vi "虛擬儀控期末專題R09543010張哲睿主程式.vi"() -> ()   [LabVIEW 2014]
uses:
  <vilib>/Math Plots/3D Math Plots/3D Pie/3D Pie XCtrl/3D Pie.xctl
  <vilib>/Math Plots/3D Math Plots/3D Pie/3D Pie Datatype/Public/Plot Helper (Vector).vi
  <vilib>/Math Plots/3D Math Plots/3D Pie/3D Pie Datatype/3D Pie Datatype.lvclass
panel:
  in  "再感染機率":dbl=20.0 format="%#_13g%%"
  out "3D Pie":refnum<class "3D Plot Datatype.lvclass">[](xcontrol)
  out "P10 Infeted":enum16{"Infected", "Uninfected"}(ring)
  out "P9 Infeted?":enum16{"Infected", "Uninfected"}(ring)
  out "P8 Infeted?":enum16{"Infected", "Uninfected"}(ring)
  out "P7 Infeted?":enum16{"Infected", "Uninfected"}(ring)
  out "P6 Infeted?":enum16{"Infected", "Uninfected"}(ring)
  out "P5 Infeted?":enum16{"Infected", "Uninfected"}(ring)
  out "P4 Infeted?":enum16{"Infected", "Uninfected"}(ring)
  out "P3 Infeted?":enum16{"Infected", "Uninfected"}(ring)
  out "P2 Infeted?":enum16{"Infected", "Uninfected"}(ring)
  out "P1 Infeted?":enum16{"Infected", "Uninfected"}(ring)
  in  "死亡率":dbl=50.0 format="%#_g%%"
  in  "陰轉陽率":dbl=50.0 format="%#_g%%"
  out "Alive? P10":enum16{"Alive", "Dead"}(ring)
  out "Alive? P9":enum16{"Alive", "Dead"}(ring)
  out "Alive? P8":enum16{"Alive", "Dead"}(ring)
  out "Alive? P7":enum16{"Alive", "Dead"}(ring)
  out "Alive? P6":enum16{"Alive", "Dead"}(ring)
  out "Alive? P5":enum16{"Alive", "Dead"}(ring)
  out "Alive? P4":enum16{"Alive", "Dead"}(ring)
  out "Alive? P3":enum16{"Alive", "Dead"}(ring)
  out "Alive? P2":enum16{"Alive", "Dead"}(ring)
  out "Alive? P1":enum16{"Alive", "Dead"}(ring)
  in  "stop":bool
  out "Y":i32[](array[numeric])
  out "X":i32[](array[numeric])
  out "Numeric":i32
  out "P1":bool
  in  "Bound right":dbl=300.0
  in  "Bound bottom":dbl=300.0
  out "State":T1(ring)
  out "P2":bool
  out "State 2":T1(ring)
  out "State 3":T1(ring)
  out "P3":bool
  out "P4":bool
  out "State 4":T1(ring)
  out "State 5":T1(ring)
  out "P5":bool
  out "State 6":T1(ring)
  out "P6":bool
  out "State 7":T1(ring)
  out "P7":bool
  out "State 8":T1(ring)
  out "State 9":T1(ring)
  out "State 10":T1(ring)
  out "P8":bool
  out "P9":bool
  out "P10":bool
  # "註:因內建3D Pie Chart的問題，偶爾打開VI時Pie Chart鐘百分比符號\n無法正常顯示，檔案重開一次即可解決問題"
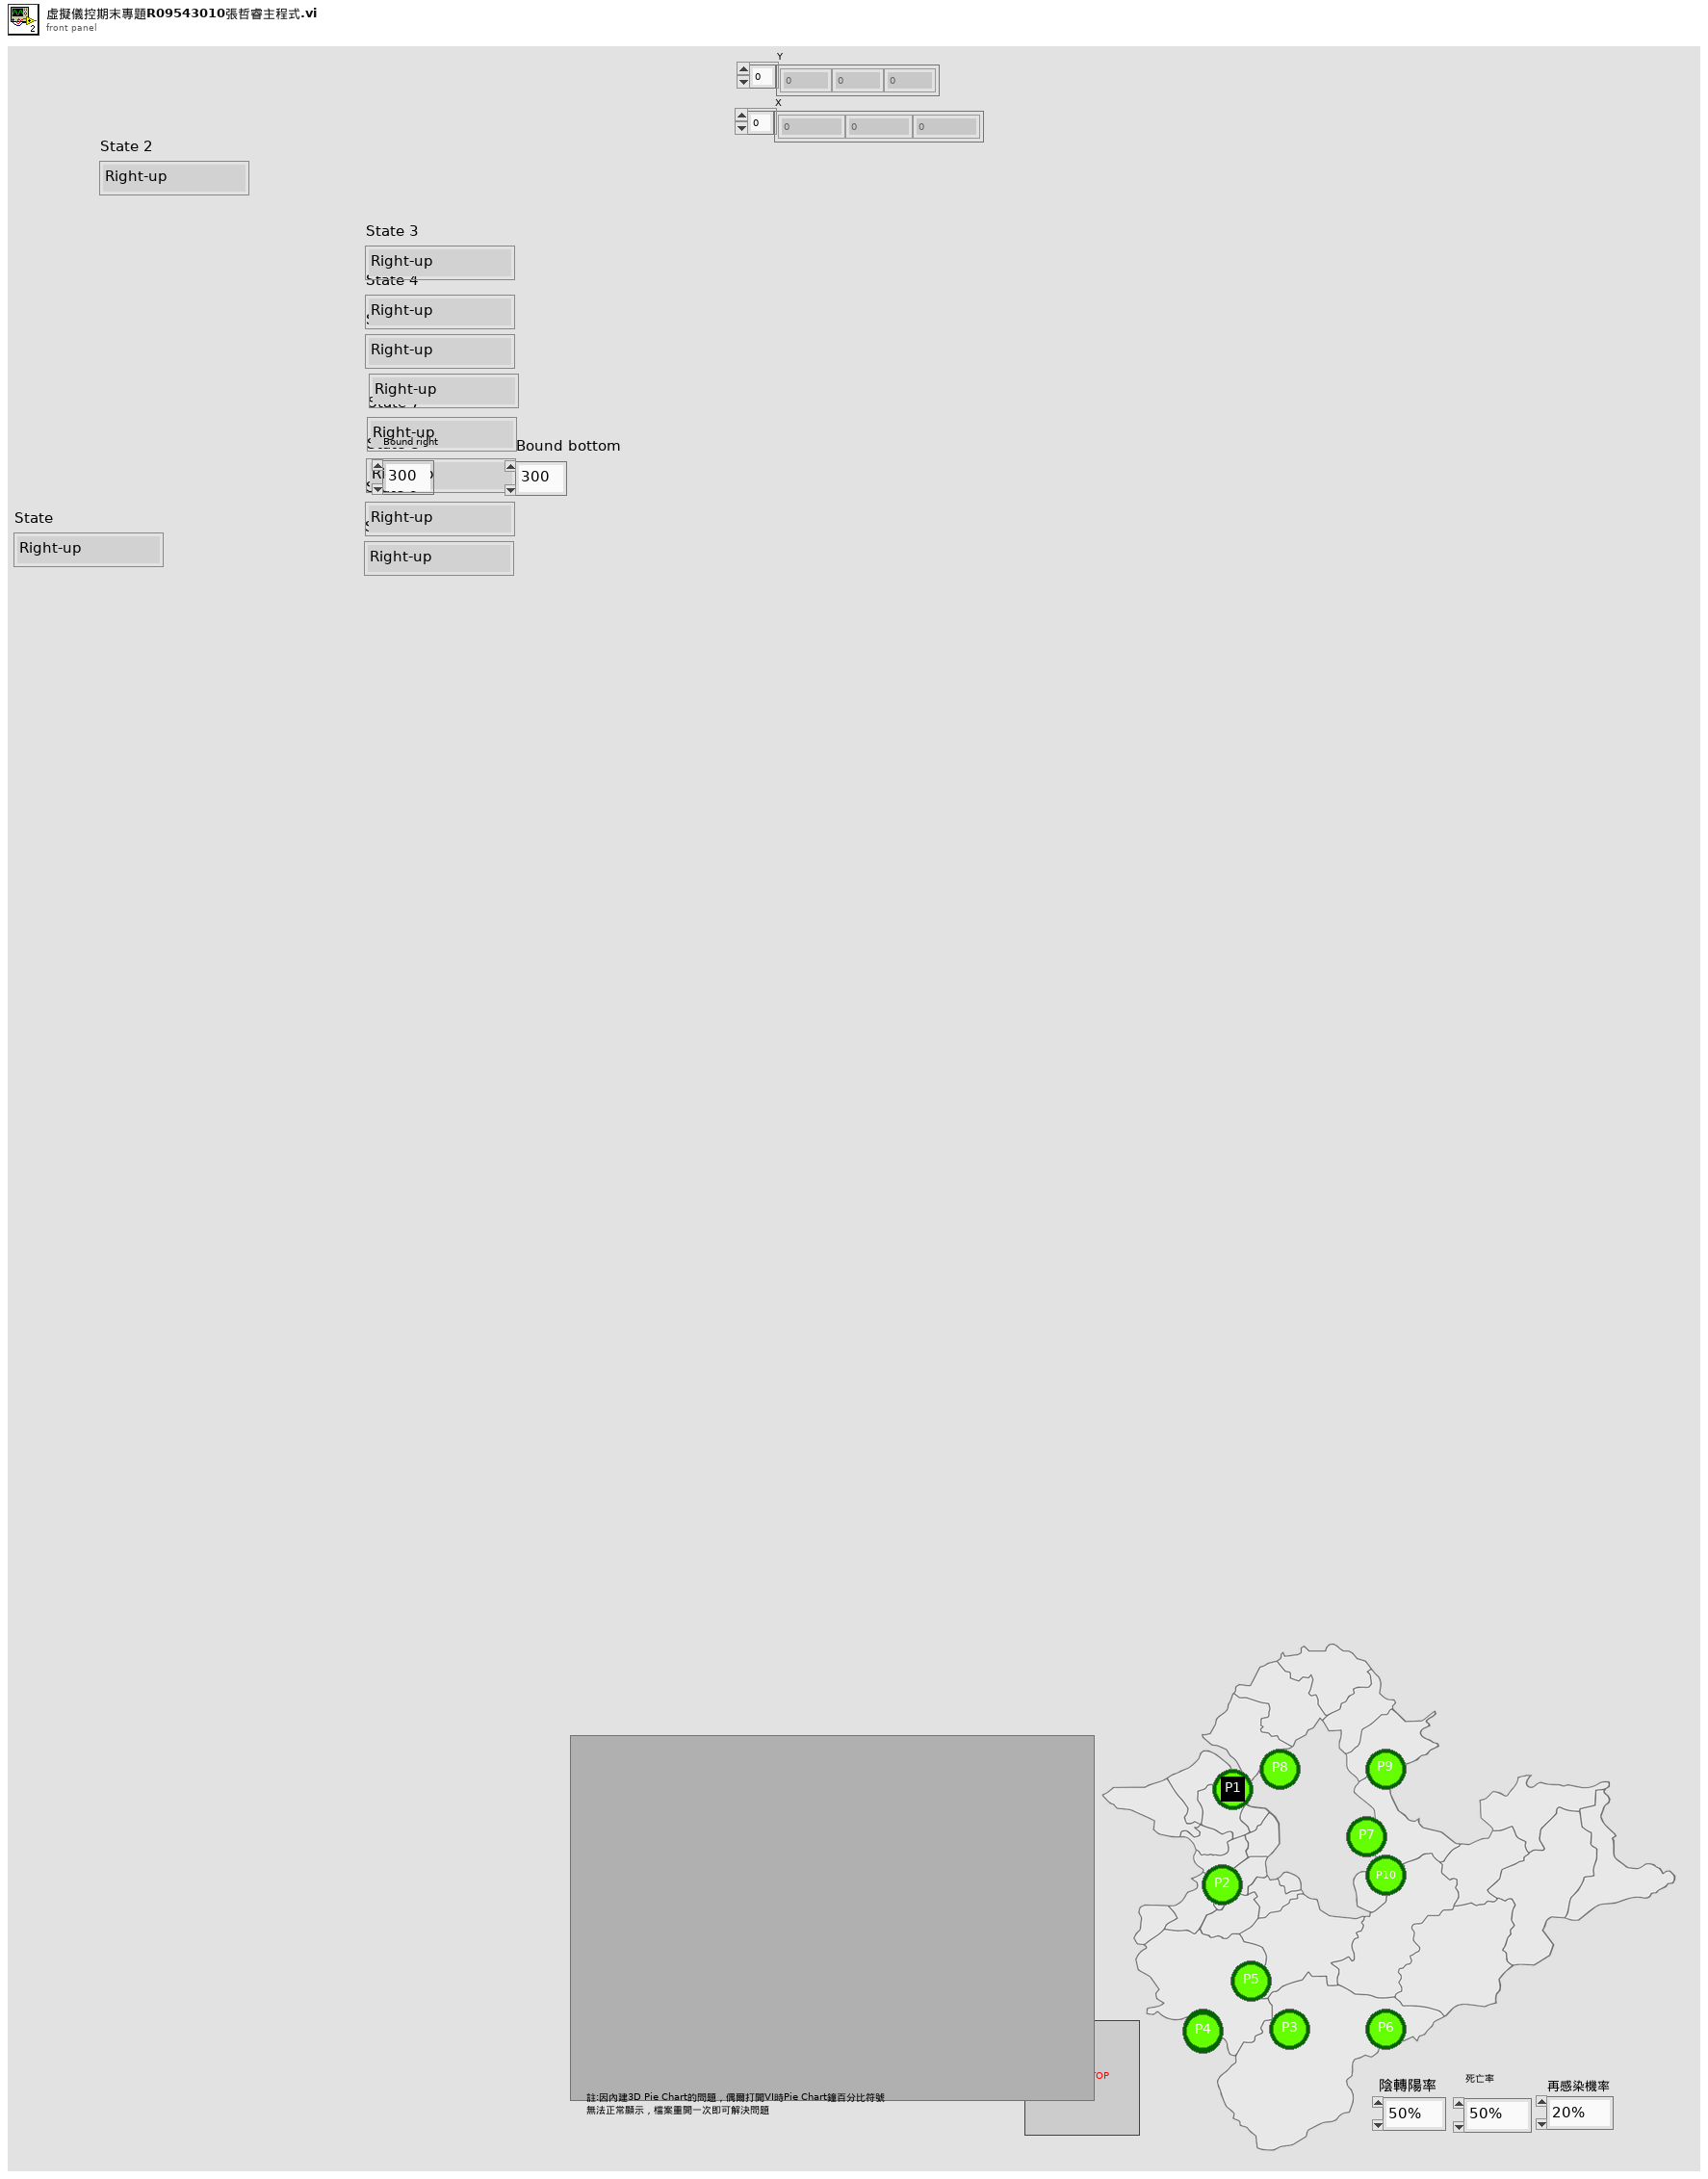
[diagram p1: front panel]
types:
  T1 = enum16{"Right-up", "Left-up", "Left-down", "Right-down"}
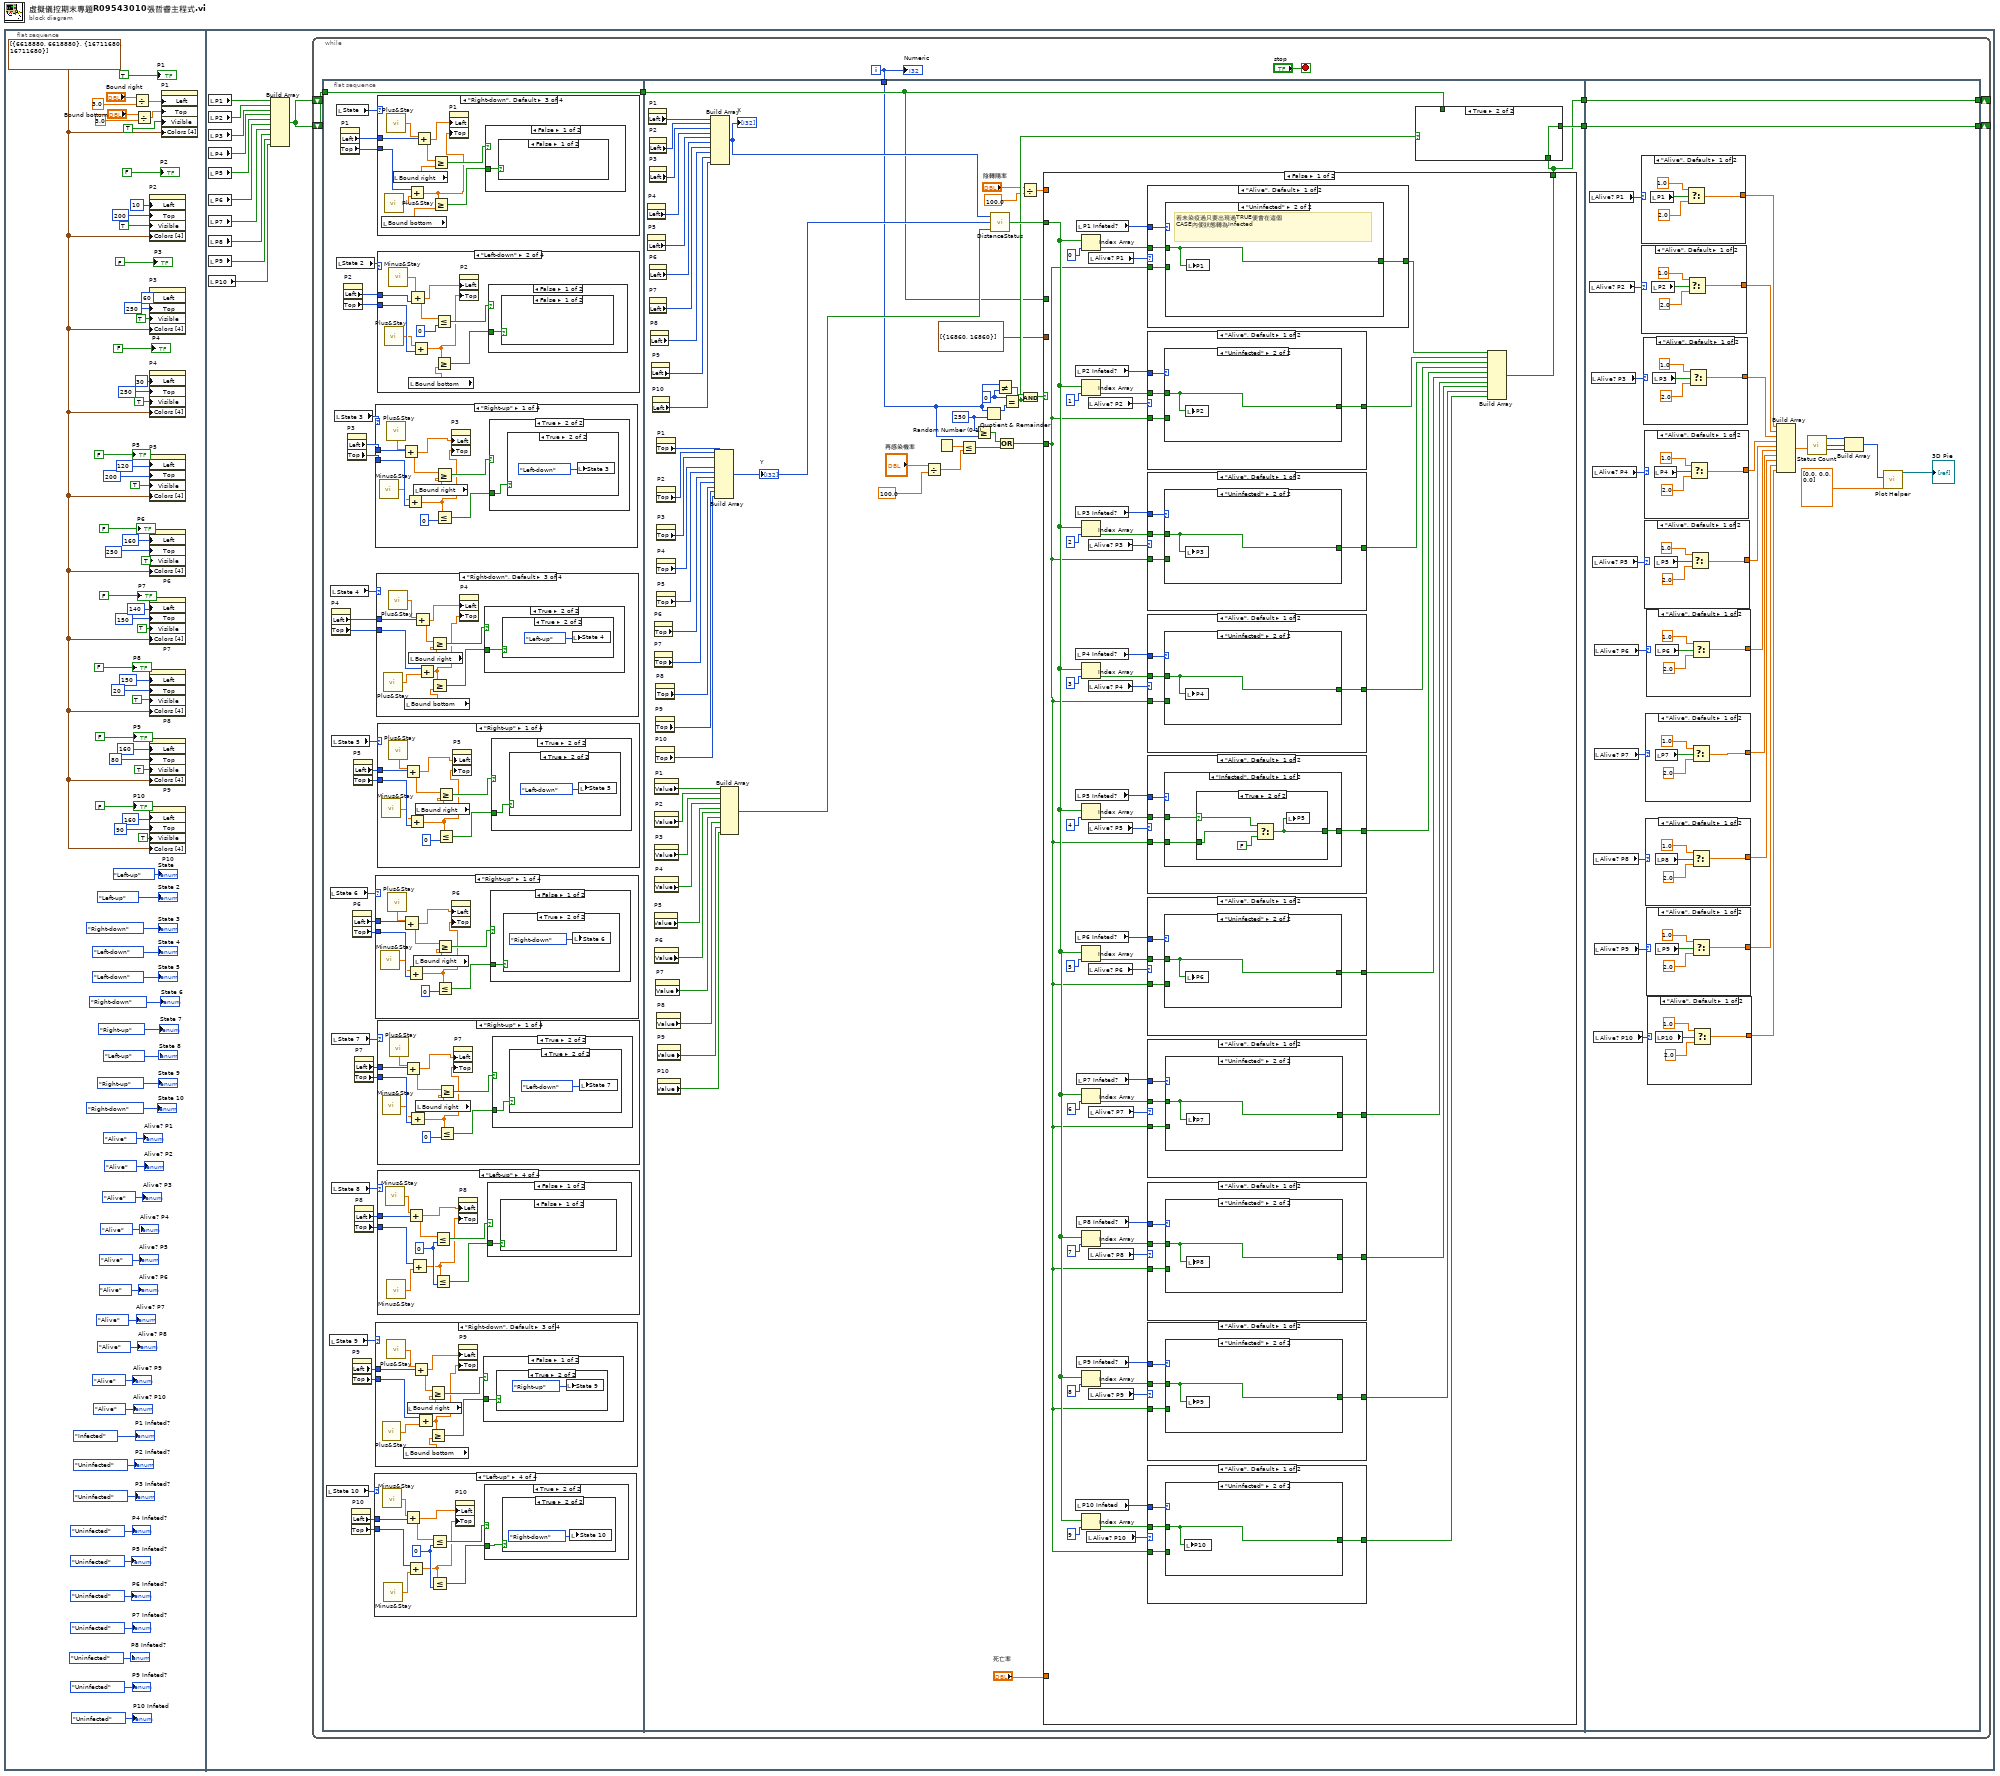
[diagram p0: block diagram]
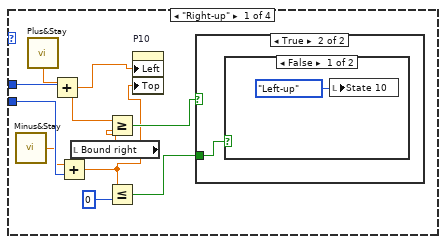
[diagram p2: hidden frame]
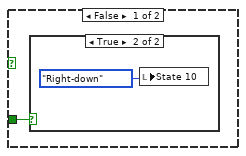
[diagram p3: hidden frame]
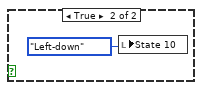
[diagram p5: hidden frame]
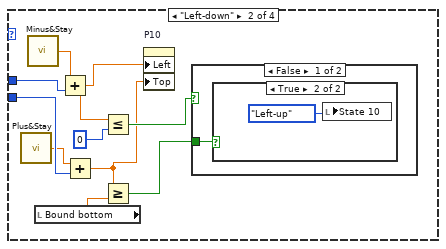
[diagram p6: hidden frame]
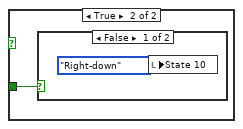
[diagram p8: hidden frame]
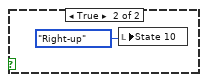
[diagram p9: hidden frame]
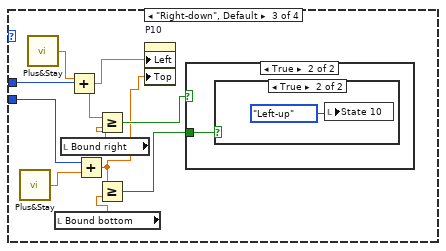
[diagram p10: hidden frame]
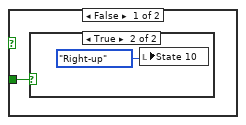
[diagram p11: hidden frame]
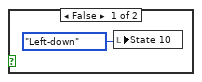
[diagram p13: hidden frame]
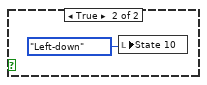
[diagram p15: hidden frame]
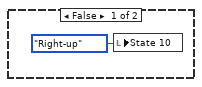
[diagram p16: hidden frame]
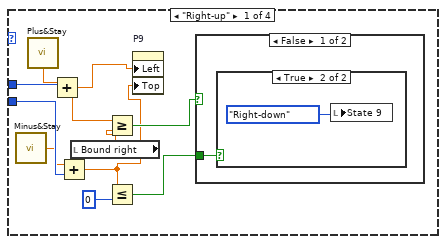
[diagram p17: hidden frame]
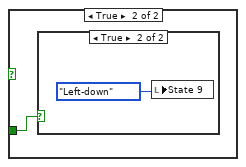
[diagram p19: hidden frame]
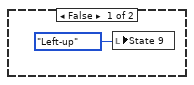
[diagram p20: hidden frame]
diagram:
  n1 = flat-sequence {
    frame #0 {
      w10 = cluster{u32, u32}[] [{6618880, 6618880}, {16711680, 16711680}] ("Colors [4]")
      n2 = Divide(x="Bound right", y=3.0) -> (x/y=w71:dbl)
      n3 = Divide(x="Bound bottom", y=3.0) -> (x/y=w70:dbl)
      n4 = property on="P2" class="Bool (strict)"("Left"=10 ("Position:Left"), "Top"=200 ("Position:Top"), "Visible"=TRUE, "Colors [4]"=w10) -> ()  [unwired: 2 in, 2 out]
      n5 = property on="P3" class="Bool (strict)"("Left"=60 ("Position:Left"), "Top"=250 ("Position:Top"), "Visible"=TRUE, "Colors [4]"=w10) -> ()  [unwired: 2 in, 2 out]
      n6 = property on="P4" class="Bool (strict)"("Left"=30 ("Position:Left"), "Top"=250 ("Position:Top"), "Visible"=TRUE, "Colors [4]"=w10) -> ()  [unwired: 2 in, 2 out]
      n7 = property on="P5" class="Bool (strict)"("Left"=120 ("Position:Left"), "Top"=200 ("Position:Top"), "Visible"=TRUE, "Colors [4]"=w10) -> ()  [unwired: 2 in, 2 out]
      n8 = property on="P6" class="Bool (strict)"("Left"=160 ("Position:Left"), "Top"=250 ("Position:Top"), "Visible"=TRUE, "Colors [4]"=w10) -> ()  [unwired: 2 in, 2 out]
      n9 = property on="P7" class="Bool (strict)"("Left"=140 ("Position:Left"), "Top"=150 ("Position:Top"), "Visible"=TRUE, "Colors [4]"=w10) -> ()  [unwired: 2 in, 2 out]
      n10 = property on="P8" class="Bool (strict)"("Left"=150 ("Position:Left"), "Top"=20 ("Position:Top"), "Visible"=TRUE, "Colors [4]"=w10) -> ()  [unwired: 2 in, 2 out]
      n11 = property on="P9" class="Bool (strict)"("Left"=160 ("Position:Left"), "Top"=80 ("Position:Top"), "Visible"=TRUE, "Colors [4]"=w10) -> ()  [unwired: 2 in, 2 out]
      n12 = property on="P10" class="Bool (strict)"("Left"=160 ("Position:Left"), "Top"=90 ("Position:Top"), "Visible"=TRUE, "Colors [4]"=w10) -> ()  [unwired: 2 in, 2 out]
      n13 = property on="P1" class="Bool (strict)"("Left"=w71, "Top"=w70, "Visible"=TRUE, "Colors [4]"=w10) -> ()  [unwired: 2 in, 2 out]
      "P1" <- TRUE
      "State" <- T1."Left-up" ("State")
      "P2" <- FALSE
      "State 2" <- T1."Left-up" ("State")
      "State 3" <- T1."Right-down" ("State")
      "P3" <- FALSE
      "P4" <- FALSE
      "State 4" <- T1."Left-down" ("State")
      "State 5" <- T1."Left-down" ("State")
      "P5" <- FALSE
      "State 6" <- T1."Right-down" ("State")
      "P6" <- FALSE
      "State 7" <- T1."Right-up" ("State")
      "P7" <- FALSE
      "State 8" <- T1."Left-up" ("State")
      "State 9" <- T1."Right-up" ("State")
      "State 10" <- T1."Right-down" ("State")
      "P8" <- FALSE
      "P9" <- FALSE
      "P10" <- FALSE
      "Alive? P1" <- enum16{"Alive", "Dead"}."Alive"
      "Alive? P2" <- enum16{"Alive", "Dead"}."Alive"
      "Alive? P3" <- enum16{"Alive", "Dead"}."Alive"
      "Alive? P4" <- enum16{"Alive", "Dead"}."Alive"
      "Alive? P5" <- enum16{"Alive", "Dead"}."Alive"
      "Alive? P6" <- enum16{"Alive", "Dead"}."Alive"
      "Alive? P7" <- enum16{"Alive", "Dead"}."Alive"
      "Alive? P8" <- enum16{"Alive", "Dead"}."Alive"
      "Alive? P9" <- enum16{"Alive", "Dead"}."Alive"
      "Alive? P10" <- enum16{"Alive", "Dead"}."Alive"
      "P1 Infeted?" <- enum16{"Infected", "Uninfected"}."Infected"
      "P2 Infeted?" <- enum16{"Infected", "Uninfected"}."Uninfected"
      "P3 Infeted?" <- enum16{"Infected", "Uninfected"}."Uninfected"
      "P4 Infeted?" <- enum16{"Infected", "Uninfected"}."Uninfected"
      "P5 Infeted?" <- enum16{"Infected", "Uninfected"}."Uninfected"
      "P6 Infeted?" <- enum16{"Infected", "Uninfected"}."Uninfected"
      "P7 Infeted?" <- enum16{"Infected", "Uninfected"}."Uninfected"
      "P8 Infeted?" <- enum16{"Infected", "Uninfected"}."Uninfected"
      "P9 Infeted?" <- enum16{"Infected", "Uninfected"}."Uninfected"
      "P10 Infeted" <- enum16{"Infected", "Uninfected"}."Uninfected"
    }
    frame #1 {
      n14 = local read "P1"() -> (w86:bool)
      n15 = local read "P2"() -> (w85:bool)
      n16 = local read "P3"() -> (w84:bool)
      n17 = local read "P4"() -> (w83:bool)
      n18 = local read "P5"() -> (w82:bool)
      n19 = local read "P6"() -> (w81:bool)
      n20 = local read "P7"() -> (w80:bool)
      n21 = local read "P8"() -> (w79:bool)
      n22 = local read "P9"() -> (w78:bool)
      n23 = local read "P10"() -> (w77:bool)
      n24 = Build Array(w86, w85, w84, w83, w82, w81, w80, w79, w78, w77) -> (w76:bool[])
      n25 = while {
        shift-right: [w93] -> _
        shift-left: w76 -> [_]
        shift-right: [w92] -> _
        shift-left: w76 -> [w91]
        i -> [w89]
        stop <- "stop" stop-if-true
        n26 = flat-sequence {
          tunnel: w91 -> [w116]
          tunnel: [w116] -> w90
          tunnel: w89 -> [w720]
          tunnel: w90 -> [w761]
          tunnel: [w760] -> w88
          tunnel: [w765] -> w87
          tunnel: [w1380] -> w92
          tunnel: [w1381] -> w93
          tunnel: w88 -> [w1381]
          tunnel: w87 -> [w1380]
          frame #0 {
            n27 = local read "State 10"() -> (w96:T1)
            n28 = local read "State 9"() -> (w99:T1)
            n29 = local read "State 6"() -> (w108:T1)
            n30 = local read "State 4"() -> (w114:T1)
            n31 = property on="P4" class="Bool (strict)"() -> ("Left"=w115:i32, "Top"=w113:i32)  [unwired: 2 in, 2 out]
            n32 = local read "State 5"() -> (w111:T1)
            n33 = local read "State 7"() -> (w105:T1)
            n34 = local read "State 8"() -> (w102:T1)
            n35 = local read "State 3"() -> (w119:T1)
            n36 = local read "State 2"() -> (w120:T1)
            n37 = local read "State"() -> (w125:T1)
            n38 = property on="P1" class="Bool (strict)"() -> ("Left"=w124:i32, "Top"=w123:i32)  [unwired: 2 in, 2 out]
            n39 = property on="P2" class="Bool (strict)"() -> ("Left"=w122:i32, "Top"=w121:i32)  [unwired: 2 in, 2 out]
            n40 = property on="P3" class="Bool (strict)"() -> ("Left"=w117:i32, "Top"=w118:i32)  [unwired: 2 in, 2 out]
            n41 = property on="P10" class="Bool (strict)"() -> ("Left"=w97:i32, "Top"=w95:i32)  [unwired: 2 in, 2 out]
            n42 = property on="P9" class="Bool (strict)"() -> ("Left"=w98:i32, "Top"=w100:i32)  [unwired: 2 in, 2 out]
            n43 = property on="P6" class="Bool (strict)"() -> ("Left"=w109:i32, "Top"=w107:i32)  [unwired: 2 in, 2 out]
            n44 = property on="P5" class="Bool (strict)"() -> ("Left"=w110:i32, "Top"=w112:i32)  [unwired: 2 in, 2 out]
            n45 = property on="P7" class="Bool (strict)"() -> ("Left"=w104:i32, "Top"=w106:i32)  [unwired: 2 in, 2 out]
            n46 = property on="P8" class="Bool (strict)"() -> ("Left"=w103:i32, "Top"=w101:i32)  [unwired: 2 in, 2 out]
            n47 = case shown="\"Left-up\"" w96 {
              tunnel: w97 -> [w132 w148 w165 w177]
              tunnel: w95 -> [w131 w147 w157 w172]
              frame "Right-up" {
                n48 = call "Minus&Stay.vi"() -> ("s? t:f"=w126:dbl)
                n49 = call "Plus&Stay.vi"() -> ("s? t:f"=w127:dbl)
                n50 = Add(x=w127, y=w132) -> (x+y=w129:dbl)
                n51 = Add(x=w126, y=w131) -> (x+y=w128:dbl)
                n52 = local read "Bound right"() -> (w135:dbl)
                n53 = Greater Or Equal?(x=w129, y=w135) -> (x >= y?=w134:bool)
                n54 = Less Or Equal?(x=w128, y=0) -> (x <= y?=w133:bool)
                n55 = property on="P10" class="Bool (strict)"("Left"=w129, "Top"=w128) -> ()  [unwired: 2 in, 2 out]
                n56 = case shown="True" w134 {
                  tunnel: w133 -> [w136 w138]
                  frame False {
                    n57 = case shown="True" w136 {
                      frame False {
                      }
                      frame True {
                        n58 = local write "State 10"(T1."Right-down" ("State")) -> ()
                      }
                    }
                  }
                  frame True {
                    n59 = case shown="False" w138 {
                      frame False {
                        n60 = local write "State 10"(T1."Left-up" ("State")) -> ()
                      }
                      frame True {
                        n61 = local write "State 10"(T1."Left-down" ("State")) -> ()
                      }
                    }
                  }
                }
              }
              frame "Left-down" {
                n62 = call "Plus&Stay.vi"() -> ("s? t:f"=w141:dbl)
                n63 = call "Minus&Stay.vi"() -> ("s? t:f"=w142:dbl)
                n64 = local read "Bound bottom"() -> (w146:dbl)
                n65 = Add(x=w142, y=w148) -> (x+y=w144:dbl)
                n66 = Add(x=w141, y=w147) -> (x+y=w143:dbl)
                n67 = Less Or Equal?(x=w144, y=0) -> (x <= y?=w150:bool)
                n68 = Greater Or Equal?(x=w143, y=w146) -> (x >= y?=w149:bool)
                n69 = property on="P10" class="Bool (strict)"("Left"=w144, "Top"=w143) -> ()  [unwired: 2 in, 2 out]
                n70 = case shown="False" w150 {
                  tunnel: w149 -> [w151 w153]
                  frame False {
                    n71 = case shown="True" w151 {
                      frame False {
                      }
                      frame True {
                        n72 = local write "State 10"(T1."Left-up" ("State")) -> ()
                      }
                    }
                  }
                  frame True {
                    n73 = case shown="False" w153 {
                      frame False {
                        n74 = local write "State 10"(T1."Right-down" ("State")) -> ()
                      }
                      frame True {
                        n75 = local write "State 10"(T1."Right-up" ("State")) -> ()
                      }
                    }
                  }
                }
              }
              frame "Right-down", Default {
                n76 = call "Plus&Stay.vi"() -> ("s? t:f"=w156:dbl)
                n77 = call "Plus&Stay.vi"() -> ("s? t:f"=w158:dbl)
                n78 = local read "Bound bottom"() -> (w163:dbl)
                n79 = local read "Bound right"() -> (w164:dbl)
                n80 = Add(x=w158, y=w165) -> (x+y=w160:dbl)
                n81 = Add(x=w157, y=w156) -> (x+y=w159:dbl)
                n82 = Greater Or Equal?(x=w160, y=w164) -> (x >= y?=w162:bool)
                n83 = Greater Or Equal?(x=w159, y=w163) -> (x >= y?=w161:bool)
                n84 = property on="P10" class="Bool (strict)"("Left"=w160, "Top"=w159) -> ()  [unwired: 2 in, 2 out]
                n85 = case shown="True" w162 {
                  tunnel: w161 -> [w166 w168]
                  frame False {
                    n86 = case shown="True" w166 {
                      frame False {
                      }
                      frame True {
                        n87 = local write "State 10"(T1."Right-up" ("State")) -> ()
                      }
                    }
                  }
                  frame True {
                    n88 = case shown="True" w168 {
                      frame False {
                        n89 = local write "State 10"(T1."Left-down" ("State")) -> ()
                      }
                      frame True {
                        n90 = local write "State 10"(T1."Left-up" ("State")) -> ()
                      }
                    }
                  }
                }
              }
              frame "Left-up" {
                w176 = 0 ("y")
                n91 = call "Minus&Stay.vi"() -> ("s? t:f"=w173:dbl)
                n92 = call "Minus&Stay.vi"() -> ("s? t:f"=w171:dbl)
                n93 = Add(x=w173, y=w177) -> (x+y=w175:dbl)
                n94 = Add(x=w172, y=w171) -> (x+y=w174:dbl)
                n95 = Less Or Equal?(x=w175, y=w176) -> (x <= y?=w179:bool)
                n96 = Less Or Equal?(x=w174, y=w176) -> (x <= y?=w178:bool)
                n97 = property on="P10" class="Bool (strict)"("Left"=w175, "Top"=w174) -> ()  [unwired: 2 in, 2 out]
                n98 = case shown="True" w179 {
                  tunnel: w178 -> [w180 w182]
                  frame False {
                    n99 = case shown="False" w180 {
                      frame False {
                      }
                      frame True {
                        n100 = local write "State 10"(T1."Left-down" ("State")) -> ()
                      }
                    }
                  }
                  frame True {
                    n101 = case shown="True" w182 {
                      frame False {
                        n102 = local write "State 10"(T1."Right-up" ("State")) -> ()
                      }
                      frame True {
                        n103 = local write "State 10"(T1."Right-down" ("State")) -> ()
                      }
                    }
                  }
                }
              }
            }
            n104 = case shown="\"Right-up\"" w119 {
              tunnel: w117 -> [w545 w561 w578 w590]
              tunnel: w118 -> [w544 w560 w570 w585]
              frame "Right-up" {
                n105 = call "Minus&Stay.vi"() -> ("s? t:f"=w539:dbl)
                n106 = call "Plus&Stay.vi"() -> ("s? t:f"=w540:dbl)
                n107 = Add(x=w540, y=w545) -> (x+y=w542:dbl)
                n108 = Add(x=w539, y=w544) -> (x+y=w541:dbl)
                n109 = local read "Bound right"() -> (w548:dbl)
                n110 = Greater Or Equal?(x=w542, y=w548) -> (x >= y?=w547:bool)
                n111 = Less Or Equal?(x=w541, y=0) -> (x <= y?=w546:bool)
                n112 = property on="P3" class="Bool (strict)"("Left"=w542, "Top"=w541) -> ()  [unwired: 2 in, 2 out]
                n113 = case shown="True" w547 {
                  tunnel: w546 -> [w549 w551]
                  frame False {
                    n114 = case shown="False" w549 {
                      frame False {
                      }
                      frame True {
                        n115 = local write "State 3"(T1."Right-down" ("State")) -> ()
                      }
                    }
                  }
                  frame True {
                    n116 = case shown="True" w551 {
                      frame False {
                        n117 = local write "State 3"(T1."Left-up" ("State")) -> ()
                      }
                      frame True {
                        n118 = local write "State 3"(T1."Left-down" ("State")) -> ()
                      }
                    }
                  }
                }
              }
              frame "Left-down" {
                n119 = call "Plus&Stay.vi"() -> ("s? t:f"=w554:dbl)
                n120 = call "Minus&Stay.vi"() -> ("s? t:f"=w555:dbl)
                n121 = local read "Bound bottom"() -> (w559:dbl)
                n122 = Add(x=w555, y=w561) -> (x+y=w557:dbl)
                n123 = Add(x=w554, y=w560) -> (x+y=w556:dbl)
                n124 = Less Or Equal?(x=w557, y=0) -> (x <= y?=w563:bool)
                n125 = Greater Or Equal?(x=w556, y=w559) -> (x >= y?=w562:bool)
                n126 = property on="P3" class="Bool (strict)"("Left"=w557, "Top"=w556) -> ()  [unwired: 2 in, 2 out]
                n127 = case shown="True" w563 {
                  tunnel: w562 -> [w564 w566]
                  frame False {
                    n128 = case shown="True" w564 {
                      frame False {
                      }
                      frame True {
                        n129 = local write "State 3"(T1."Left-up" ("State")) -> ()
                      }
                    }
                  }
                  frame True {
                    n130 = case shown="True" w566 {
                      frame False {
                        n131 = local write "State 3"(T1."Right-down" ("State")) -> ()
                      }
                      frame True {
                        n132 = local write "State 3"(T1."Right-up" ("State")) -> ()
                      }
                    }
                  }
                }
              }
              frame "Right-down", Default {
                n133 = call "Plus&Stay.vi"() -> ("s? t:f"=w569:dbl)
                n134 = call "Plus&Stay.vi"() -> ("s? t:f"=w571:dbl)
                n135 = local read "Bound bottom"() -> (w576:dbl)
                n136 = local read "Bound right"() -> (w577:dbl)
                n137 = Add(x=w571, y=w578) -> (x+y=w573:dbl)
                n138 = Add(x=w570, y=w569) -> (x+y=w572:dbl)
                n139 = Greater Or Equal?(x=w573, y=w577) -> (x >= y?=w575:bool)
                n140 = Greater Or Equal?(x=w572, y=w576) -> (x >= y?=w574:bool)
                n141 = property on="P3" class="Bool (strict)"("Left"=w573, "Top"=w572) -> ()  [unwired: 2 in, 2 out]
                n142 = case shown="False" w575 {
                  tunnel: w574 -> [w579 w581]
                  frame False {
                    n143 = case shown="False" w579 {
                      frame False {
                      }
                      frame True {
                        n144 = local write "State 3"(T1."Right-up" ("State")) -> ()
                      }
                    }
                  }
                  frame True {
                    n145 = case shown="False" w581 {
                      frame False {
                        n146 = local write "State 3"(T1."Left-down" ("State")) -> ()
                      }
                      frame True {
                        n147 = local write "State 3"(T1."Left-up" ("State")) -> ()
                      }
                    }
                  }
                }
              }
              frame "Left-up" {
                w589 = 0 ("y")
                n148 = call "Minus&Stay.vi"() -> ("s? t:f"=w586:dbl)
                n149 = call "Minus&Stay.vi"() -> ("s? t:f"=w584:dbl)
                n150 = Add(x=w586, y=w590) -> (x+y=w588:dbl)
                n151 = Add(x=w585, y=w584) -> (x+y=w587:dbl)
                n152 = Less Or Equal?(x=w588, y=w589) -> (x <= y?=w592:bool)
                n153 = Less Or Equal?(x=w587, y=w589) -> (x <= y?=w591:bool)
                n154 = property on="P3" class="Bool (strict)"("Left"=w588, "Top"=w587) -> ()  [unwired: 2 in, 2 out]
                n155 = case shown="False" w592 {
                  tunnel: w591 -> [w593 w595]
                  frame False {
                    n156 = case shown="True" w593 {
                      frame False {
                      }
                      frame True {
                        n157 = local write "State 3"(T1."Left-down" ("State")) -> ()
                      }
                    }
                  }
                  frame True {
                    n158 = case shown="False" w595 {
                      frame False {
                        n159 = local write "State 3"(T1."Right-up" ("State")) -> ()
                      }
                      frame True {
                        n160 = local write "State 3"(T1."Right-down" ("State")) -> ()
                      }
                    }
                  }
                }
              }
            }
            n161 = case shown="\"Right-down\", Default" w99 {
              tunnel: w98 -> [w191 w207 w224 w236]
              tunnel: w100 -> [w190 w206 w216 w231]
              frame "Right-up" {
                n162 = call "Minus&Stay.vi"() -> ("s? t:f"=w185:dbl)
                n163 = call "Plus&Stay.vi"() -> ("s? t:f"=w186:dbl)
                n164 = Add(x=w186, y=w191) -> (x+y=w188:dbl)
                n165 = Add(x=w185, y=w190) -> (x+y=w187:dbl)
                n166 = local read "Bound right"() -> (w194:dbl)
                n167 = Greater Or Equal?(x=w188, y=w194) -> (x >= y?=w193:bool)
                n168 = Less Or Equal?(x=w187, y=0) -> (x <= y?=w192:bool)
                n169 = property on="P9" class="Bool (strict)"("Left"=w188, "Top"=w187) -> ()  [unwired: 2 in, 2 out]
                n170 = case shown="False" w193 {
                  tunnel: w192 -> [w195 w197]
                  frame False {
                    n171 = case shown="True" w195 {
                      frame False {
                      }
                      frame True {
                        n172 = local write "State 9"(T1."Right-down" ("State")) -> ()
                      }
                    }
                  }
                  frame True {
                    n173 = case shown="True" w197 {
                      frame False {
                        n174 = local write "State 9"(T1."Left-up" ("State")) -> ()
                      }
                      frame True {
                        n175 = local write "State 9"(T1."Left-down" ("State")) -> ()
                      }
                    }
                  }
                }
              }
              frame "Left-down" {
                n176 = call "Plus&Stay.vi"() -> ("s? t:f"=w200:dbl)
                n177 = call "Minus&Stay.vi"() -> ("s? t:f"=w201:dbl)
                n178 = local read "Bound bottom"() -> (w205:dbl)
                n179 = Add(x=w201, y=w207) -> (x+y=w203:dbl)
                n180 = Add(x=w200, y=w206) -> (x+y=w202:dbl)
                n181 = Less Or Equal?(x=w203, y=0) -> (x <= y?=w209:bool)
                n182 = Greater Or Equal?(x=w202, y=w205) -> (x >= y?=w208:bool)
                n183 = property on="P9" class="Bool (strict)"("Left"=w203, "Top"=w202) -> ()  [unwired: 2 in, 2 out]
                n184 = case shown="True" w209 {
                  tunnel: w208 -> [w210 w212]
                  frame False {
                    n185 = case shown="True" w210 {
                      frame False {
                      }
                      frame True {
                        n186 = local write "State 9"(T1."Left-up" ("State")) -> ()
                      }
                    }
                  }
                  frame True {
                    n187 = case shown="True" w212 {
                      frame False {
                        n188 = local write "State 9"(T1."Right-down" ("State")) -> ()
                      }
                      frame True {
                        n189 = local write "State 9"(T1."Right-up" ("State")) -> ()
                      }
                    }
                  }
                }
              }
              frame "Right-down", Default {
                n190 = call "Plus&Stay.vi"() -> ("s? t:f"=w215:dbl)
                n191 = call "Plus&Stay.vi"() -> ("s? t:f"=w217:dbl)
                n192 = local read "Bound bottom"() -> (w222:dbl)
                n193 = local read "Bound right"() -> (w223:dbl)
                n194 = Add(x=w217, y=w224) -> (x+y=w219:dbl)
                n195 = Add(x=w216, y=w215) -> (x+y=w218:dbl)
                n196 = Greater Or Equal?(x=w219, y=w223) -> (x >= y?=w221:bool)
                n197 = Greater Or Equal?(x=w218, y=w222) -> (x >= y?=w220:bool)
                n198 = property on="P9" class="Bool (strict)"("Left"=w219, "Top"=w218) -> ()  [unwired: 2 in, 2 out]
                n199 = case shown="False" w221 {
                  tunnel: w220 -> [w225 w227]
                  frame False {
                    n200 = case shown="True" w225 {
                      frame False {
                      }
                      frame True {
                        n201 = local write "State 9"(T1."Right-up" ("State")) -> ()
                      }
                    }
                  }
                  frame True {
                    n202 = case shown="False" w227 {
                      frame False {
                        n203 = local write "State 9"(T1."Left-down" ("State")) -> ()
                      }
                      frame True {
                        n204 = local write "State 9"(T1."Left-up" ("State")) -> ()
                      }
                    }
                  }
                }
              }
              frame "Left-up" {
                w235 = 0 ("y")
                n205 = call "Minus&Stay.vi"() -> ("s? t:f"=w232:dbl)
                n206 = call "Minus&Stay.vi"() -> ("s? t:f"=w230:dbl)
                n207 = Add(x=w232, y=w236) -> (x+y=w234:dbl)
                n208 = Add(x=w231, y=w230) -> (x+y=w233:dbl)
                n209 = Less Or Equal?(x=w234, y=w235) -> (x <= y?=w238:bool)
                n210 = Less Or Equal?(x=w233, y=w235) -> (x <= y?=w237:bool)
                n211 = property on="P9" class="Bool (strict)"("Left"=w234, "Top"=w233) -> ()  [unwired: 2 in, 2 out]
                n212 = case shown="False" w238 {
                  tunnel: w237 -> [w239 w241]
                  frame False {
                    n213 = case shown="True" w239 {
                      frame False {
                      }
                      frame True {
                        n214 = local write "State 9"(T1."Left-down" ("State")) -> ()
                      }
                    }
                  }
                  frame True {
                    n215 = case shown="True" w241 {
                      frame False {
                        n216 = local write "State 9"(T1."Right-up" ("State")) -> ()
                      }
                      frame True {
                        n217 = local write "State 9"(T1."Right-down" ("State")) -> ()
                      }
                    }
                  }
                }
              }
            }
            n218 = case shown="\"Right-up\"" w108 {
              tunnel: w109 -> [w368 w384 w401 w413]
              tunnel: w107 -> [w367 w383 w393 w408]
              frame "Right-up" {
                n219 = call "Minus&Stay.vi"() -> ("s? t:f"=w362:dbl)
                n220 = call "Plus&Stay.vi"() -> ("s? t:f"=w363:dbl)
                n221 = Add(x=w363, y=w368) -> (x+y=w365:dbl)
                n222 = Add(x=w362, y=w367) -> (x+y=w364:dbl)
                n223 = local read "Bound right"() -> (w371:dbl)
                n224 = Greater Or Equal?(x=w365, y=w371) -> (x >= y?=w370:bool)
                n225 = Less Or Equal?(x=w364, y=0) -> (x <= y?=w369:bool)
                n226 = property on="P6" class="Bool (strict)"("Left"=w365, "Top"=w364) -> ()  [unwired: 2 in, 2 out]
                n227 = case shown="False" w370 {
                  tunnel: w369 -> [w372 w374]
                  frame False {
                    n228 = case shown="True" w372 {
                      frame False {
                      }
                      frame True {
                        n229 = local write "State 6"(T1."Right-down" ("State")) -> ()
                      }
                    }
                  }
                  frame True {
                    n230 = case shown="False" w374 {
                      frame False {
                        n231 = local write "State 6"(T1."Left-up" ("State")) -> ()
                      }
                      frame True {
                        n232 = local write "State 6"(T1."Left-down" ("State")) -> ()
                      }
                    }
                  }
                }
              }
              frame "Left-down" {
                n233 = call "Plus&Stay.vi"() -> ("s? t:f"=w377:dbl)
                n234 = call "Minus&Stay.vi"() -> ("s? t:f"=w378:dbl)
                n235 = local read "Bound bottom"() -> (w382:dbl)
                n236 = Add(x=w378, y=w384) -> (x+y=w380:dbl)
                n237 = Add(x=w377, y=w383) -> (x+y=w379:dbl)
                n238 = Less Or Equal?(x=w380, y=0) -> (x <= y?=w386:bool)
                n239 = Greater Or Equal?(x=w379, y=w382) -> (x >= y?=w385:bool)
                n240 = property on="P6" class="Bool (strict)"("Left"=w380, "Top"=w379) -> ()  [unwired: 2 in, 2 out]
                n241 = case shown="False" w386 {
                  tunnel: w385 -> [w387 w389]
                  frame False {
                    n242 = case shown="True" w387 {
                      frame False {
                      }
                      frame True {
                        n243 = local write "State 6"(T1."Left-up" ("State")) -> ()
                      }
                    }
                  }
                  frame True {
                    n244 = case shown="False" w389 {
                      frame False {
                        n245 = local write "State 6"(T1."Right-down" ("State")) -> ()
                      }
                      frame True {
                        n246 = local write "State 6"(T1."Right-up" ("State")) -> ()
                      }
                    }
                  }
                }
              }
              frame "Right-down", Default {
                n247 = call "Plus&Stay.vi"() -> ("s? t:f"=w392:dbl)
                n248 = call "Plus&Stay.vi"() -> ("s? t:f"=w394:dbl)
                n249 = local read "Bound bottom"() -> (w399:dbl)
                n250 = local read "Bound right"() -> (w400:dbl)
                n251 = Add(x=w394, y=w401) -> (x+y=w396:dbl)
                n252 = Add(x=w393, y=w392) -> (x+y=w395:dbl)
                n253 = Greater Or Equal?(x=w396, y=w400) -> (x >= y?=w398:bool)
                n254 = Greater Or Equal?(x=w395, y=w399) -> (x >= y?=w397:bool)
                n255 = property on="P6" class="Bool (strict)"("Left"=w396, "Top"=w395) -> ()  [unwired: 2 in, 2 out]
                n256 = case shown="False" w398 {
                  tunnel: w397 -> [w402 w404]
                  frame False {
                    n257 = case shown="True" w402 {
                      frame False {
                      }
                      frame True {
                        n258 = local write "State 6"(T1."Right-up" ("State")) -> ()
                      }
                    }
                  }
                  frame True {
                    n259 = case shown="True" w404 {
                      frame False {
                        n260 = local write "State 6"(T1."Left-down" ("State")) -> ()
                      }
                      frame True {
                        n261 = local write "State 6"(T1."Left-up" ("State")) -> ()
                      }
                    }
                  }
                }
              }
              frame "Left-up" {
                w412 = 0 ("y")
                n262 = call "Minus&Stay.vi"() -> ("s? t:f"=w409:dbl)
                n263 = call "Minus&Stay.vi"() -> ("s? t:f"=w407:dbl)
                n264 = Add(x=w409, y=w413) -> (x+y=w411:dbl)
                n265 = Add(x=w408, y=w407) -> (x+y=w410:dbl)
                n266 = Less Or Equal?(x=w411, y=w412) -> (x <= y?=w415:bool)
                n267 = Less Or Equal?(x=w410, y=w412) -> (x <= y?=w414:bool)
                n268 = property on="P6" class="Bool (strict)"("Left"=w411, "Top"=w410) -> ()  [unwired: 2 in, 2 out]
                n269 = case shown="True" w415 {
                  tunnel: w414 -> [w416 w418]
                  frame False {
                    n270 = case shown="True" w416 {
                      frame False {
                      }
                      frame True {
                        n271 = local write "State 6"(T1."Left-down" ("State")) -> ()
                      }
                    }
                  }
                  frame True {
                    n272 = case shown="False" w418 {
                      frame False {
                        n273 = local write "State 6"(T1."Right-up" ("State")) -> ()
                      }
                      frame True {
                        n274 = local write "State 6"(T1."Right-down" ("State")) -> ()
                      }
                    }
                  }
                }
              }
            }
            n275 = case shown="\"Right-down\", Default" w114 {
              tunnel: w115 -> [w486 w502 w519 w531]
              tunnel: w113 -> [w485 w501 w511 w526]
              frame "Right-up" {
                n276 = call "Minus&Stay.vi"() -> ("s? t:f"=w480:dbl)
                n277 = call "Plus&Stay.vi"() -> ("s? t:f"=w481:dbl)
                n278 = Add(x=w481, y=w486) -> (x+y=w483:dbl)
                n279 = Add(x=w480, y=w485) -> (x+y=w482:dbl)
                n280 = local read "Bound right"() -> (w489:dbl)
                n281 = Greater Or Equal?(x=w483, y=w489) -> (x >= y?=w488:bool)
                n282 = Less Or Equal?(x=w482, y=0) -> (x <= y?=w487:bool)
                n283 = property on="P4" class="Bool (strict)"("Left"=w483, "Top"=w482) -> ()  [unwired: 2 in, 2 out]
                n284 = case shown="True" w488 {
                  tunnel: w487 -> [w490 w492]
                  frame False {
                    n285 = case shown="True" w490 {
                      frame False {
                      }
                      frame True {
                        n286 = local write "State 4"(T1."Right-down" ("State")) -> ()
                      }
                    }
                  }
                  frame True {
                    n287 = case shown="False" w492 {
                      frame False {
                        n288 = local write "State 4"(T1."Left-up" ("State")) -> ()
                      }
                      frame True {
                        n289 = local write "State 4"(T1."Left-down" ("State")) -> ()
                      }
                    }
                  }
                }
              }
              frame "Left-down" {
                n290 = call "Plus&Stay.vi"() -> ("s? t:f"=w495:dbl)
                n291 = call "Minus&Stay.vi"() -> ("s? t:f"=w496:dbl)
                n292 = local read "Bound bottom"() -> (w500:dbl)
                n293 = Add(x=w496, y=w502) -> (x+y=w498:dbl)
                n294 = Add(x=w495, y=w501) -> (x+y=w497:dbl)
                n295 = Less Or Equal?(x=w498, y=0) -> (x <= y?=w504:bool)
                n296 = Greater Or Equal?(x=w497, y=w500) -> (x >= y?=w503:bool)
                n297 = property on="P4" class="Bool (strict)"("Left"=w498, "Top"=w497) -> ()  [unwired: 2 in, 2 out]
                n298 = case shown="False" w504 {
                  tunnel: w503 -> [w505 w507]
                  frame False {
                    n299 = case shown="False" w505 {
                      frame False {
                      }
                      frame True {
                        n300 = local write "State 4"(T1."Left-up" ("State")) -> ()
                      }
                    }
                  }
                  frame True {
                    n301 = case shown="False" w507 {
                      frame False {
                        n302 = local write "State 4"(T1."Right-down" ("State")) -> ()
                      }
                      frame True {
                        n303 = local write "State 4"(T1."Right-up" ("State")) -> ()
                      }
                    }
                  }
                }
              }
              frame "Right-down", Default {
                n304 = call "Plus&Stay.vi"() -> ("s? t:f"=w510:dbl)
                n305 = call "Plus&Stay.vi"() -> ("s? t:f"=w512:dbl)
                n306 = local read "Bound bottom"() -> (w517:dbl)
                n307 = local read "Bound right"() -> (w518:dbl)
                n308 = Add(x=w512, y=w519) -> (x+y=w514:dbl)
                n309 = Add(x=w511, y=w510) -> (x+y=w513:dbl)
                n310 = Greater Or Equal?(x=w514, y=w518) -> (x >= y?=w516:bool)
                n311 = Greater Or Equal?(x=w513, y=w517) -> (x >= y?=w515:bool)
                n312 = property on="P4" class="Bool (strict)"("Left"=w514, "Top"=w513) -> ()  [unwired: 2 in, 2 out]
                n313 = case shown="True" w516 {
                  tunnel: w515 -> [w520 w522]
                  frame False {
                    n314 = case shown="True" w520 {
                      frame False {
                      }
                      frame True {
                        n315 = local write "State 4"(T1."Right-up" ("State")) -> ()
                      }
                    }
                  }
                  frame True {
                    n316 = case shown="True" w522 {
                      frame False {
                        n317 = local write "State 4"(T1."Left-down" ("State")) -> ()
                      }
                      frame True {
                        n318 = local write "State 4"(T1."Left-up" ("State")) -> ()
                      }
                    }
                  }
                }
              }
              frame "Left-up" {
                w530 = 0 ("y")
                n319 = call "Minus&Stay.vi"() -> ("s? t:f"=w527:dbl)
                n320 = call "Minus&Stay.vi"() -> ("s? t:f"=w525:dbl)
                n321 = Add(x=w527, y=w531) -> (x+y=w529:dbl)
                n322 = Add(x=w526, y=w525) -> (x+y=w528:dbl)
                n323 = Less Or Equal?(x=w529, y=w530) -> (x <= y?=w533:bool)
                n324 = Less Or Equal?(x=w528, y=w530) -> (x <= y?=w532:bool)
                n325 = property on="P4" class="Bool (strict)"("Left"=w529, "Top"=w528) -> ()  [unwired: 2 in, 2 out]
                n326 = case shown="True" w533 {
                  tunnel: w532 -> [w534 w536]
                  frame False {
                    n327 = case shown="True" w534 {
                      frame False {
                      }
                      frame True {
                        n328 = local write "State 4"(T1."Left-down" ("State")) -> ()
                      }
                    }
                  }
                  frame True {
                    n329 = case shown="True" w536 {
                      frame False {
                        n330 = local write "State 4"(T1."Right-up" ("State")) -> ()
                      }
                      frame True {
                        n331 = local write "State 4"(T1."Right-down" ("State")) -> ()
                      }
                    }
                  }
                }
              }
            }
            n332 = case shown="\"Left-down\"" w120 {
              tunnel: w122 -> [w604 w620 w637 w649]
              tunnel: w121 -> [w603 w619 w629 w644]
              frame "Right-up" {
                n333 = call "Minus&Stay.vi"() -> ("s? t:f"=w598:dbl)
                n334 = call "Plus&Stay.vi"() -> ("s? t:f"=w599:dbl)
                n335 = Add(x=w599, y=w604) -> (x+y=w601:dbl)
                n336 = Add(x=w598, y=w603) -> (x+y=w600:dbl)
                n337 = local read "Bound right"() -> (w607:dbl)
                n338 = Greater Or Equal?(x=w601, y=w607) -> (x >= y?=w606:bool)
                n339 = Less Or Equal?(x=w600, y=0) -> (x <= y?=w605:bool)
                n340 = property on="P2" class="Bool (strict)"("Left"=w601, "Top"=w600) -> ()  [unwired: 2 in, 2 out]
                n341 = case shown="False" w606 {
                  tunnel: w605 -> [w608 w610]
                  frame False {
                    n342 = case shown="True" w608 {
                      frame False {
                      }
                      frame True {
                        n343 = local write "State 2"(T1."Right-down" ("State")) -> ()
                      }
                    }
                  }
                  frame True {
                    n344 = case shown="True" w610 {
                      frame False {
                        n345 = local write "State 2"(T1."Left-up" ("State")) -> ()
                      }
                      frame True {
                        n346 = local write "State 2"(T1."Left-down" ("State")) -> ()
                      }
                    }
                  }
                }
              }
              frame "Left-down" {
                n347 = call "Plus&Stay.vi"() -> ("s? t:f"=w613:dbl)
                n348 = call "Minus&Stay.vi"() -> ("s? t:f"=w614:dbl)
                n349 = Add(x=w614, y=w620) -> (x+y=w616:dbl)
                n350 = local read "Bound bottom"() -> (w618:dbl)
                n351 = Add(x=w613, y=w619) -> (x+y=w615:dbl)
                n352 = Less Or Equal?(x=w616, y=0) -> (x <= y?=w622:bool)
                n353 = Greater Or Equal?(x=w615, y=w618) -> (x >= y?=w621:bool)
                n354 = property on="P2" class="Bool (strict)"("Left"=w616, "Top"=w615) -> ()  [unwired: 2 in, 2 out]
                n355 = case shown="False" w622 {
                  tunnel: w621 -> [w623 w625]
                  frame False {
                    n356 = case shown="False" w623 {
                      frame False {
                      }
                      frame True {
                        n357 = local write "State 2"(T1."Left-up" ("State")) -> ()
                      }
                    }
                  }
                  frame True {
                    n358 = case shown="True" w625 {
                      frame False {
                        n359 = local write "State 2"(T1."Right-down" ("State")) -> ()
                      }
                      frame True {
                        n360 = local write "State 2"(T1."Right-up" ("State")) -> ()
                      }
                    }
                  }
                }
              }
              frame "Right-down", Default {
                n361 = call "Plus&Stay.vi"() -> ("s? t:f"=w628:dbl)
                n362 = call "Plus&Stay.vi"() -> ("s? t:f"=w630:dbl)
                n363 = local read "Bound bottom"() -> (w635:dbl)
                n364 = local read "Bound right"() -> (w636:dbl)
                n365 = Add(x=w630, y=w637) -> (x+y=w632:dbl)
                n366 = Add(x=w629, y=w628) -> (x+y=w631:dbl)
                n367 = Greater Or Equal?(x=w632, y=w636) -> (x >= y?=w634:bool)
                n368 = Greater Or Equal?(x=w631, y=w635) -> (x >= y?=w633:bool)
                n369 = property on="P2" class="Bool (strict)"("Left"=w632, "Top"=w631) -> ()  [unwired: 2 in, 2 out]
                n370 = case shown="False" w634 {
                  tunnel: w633 -> [w638 w640]
                  frame False {
                    n371 = case shown="True" w638 {
                      frame False {
                      }
                      frame True {
                        n372 = local write "State 2"(T1."Right-up" ("State")) -> ()
                      }
                    }
                  }
                  frame True {
                    n373 = case shown="True" w640 {
                      frame False {
                        n374 = local write "State 2"(T1."Left-down" ("State")) -> ()
                      }
                      frame True {
                        n375 = local write "State 2"(T1."Left-up" ("State")) -> ()
                      }
                    }
                  }
                }
              }
              frame "Left-up" {
                w648 = 0 ("y")
                n376 = call "Minus&Stay.vi"() -> ("s? t:f"=w645:dbl)
                n377 = call "Minus&Stay.vi"() -> ("s? t:f"=w643:dbl)
                n378 = Add(x=w645, y=w649) -> (x+y=w647:dbl)
                n379 = Add(x=w644, y=w643) -> (x+y=w646:dbl)
                n380 = Less Or Equal?(x=w647, y=w648) -> (x <= y?=w651:bool)
                n381 = Less Or Equal?(x=w646, y=w648) -> (x <= y?=w650:bool)
                n382 = property on="P2" class="Bool (strict)"("Left"=w647, "Top"=w646) -> ()  [unwired: 2 in, 2 out]
                n383 = case shown="False" w651 {
                  tunnel: w650 -> [w652 w654]
                  frame False {
                    n384 = case shown="False" w652 {
                      frame False {
                      }
                      frame True {
                        n385 = local write "State 2"(T1."Left-down" ("State")) -> ()
                      }
                    }
                  }
                  frame True {
                    n386 = case shown="True" w654 {
                      frame False {
                        n387 = local write "State 2"(T1."Right-up" ("State")) -> ()
                      }
                      frame True {
                        n388 = local write "State 2"(T1."Right-down" ("State")) -> ()
                      }
                    }
                  }
                }
              }
            }
            n389 = case shown="\"Right-up\"" w111 {
              tunnel: w110 -> [w427 w443 w460 w472]
              tunnel: w112 -> [w426 w442 w452 w467]
              frame "Right-up" {
                n390 = call "Minus&Stay.vi"() -> ("s? t:f"=w421:dbl)
                n391 = call "Plus&Stay.vi"() -> ("s? t:f"=w422:dbl)
                n392 = Add(x=w422, y=w427) -> (x+y=w424:dbl)
                n393 = Add(x=w421, y=w426) -> (x+y=w423:dbl)
                n394 = local read "Bound right"() -> (w430:dbl)
                n395 = Greater Or Equal?(x=w424, y=w430) -> (x >= y?=w429:bool)
                n396 = Less Or Equal?(x=w423, y=0) -> (x <= y?=w428:bool)
                n397 = property on="P5" class="Bool (strict)"("Left"=w424, "Top"=w423) -> ()  [unwired: 2 in, 2 out]
                n398 = case shown="True" w429 {
                  tunnel: w428 -> [w431 w433]
                  frame False {
                    n399 = case shown="True" w431 {
                      frame False {
                      }
                      frame True {
                        n400 = local write "State 5"(T1."Right-down" ("State")) -> ()
                      }
                    }
                  }
                  frame True {
                    n401 = case shown="True" w433 {
                      frame False {
                        n402 = local write "State 5"(T1."Left-up" ("State")) -> ()
                      }
                      frame True {
                        n403 = local write "State 5"(T1."Left-down" ("State")) -> ()
                      }
                    }
                  }
                }
              }
              frame "Left-down" {
                n404 = call "Plus&Stay.vi"() -> ("s? t:f"=w436:dbl)
                n405 = call "Minus&Stay.vi"() -> ("s? t:f"=w437:dbl)
                n406 = local read "Bound bottom"() -> (w441:dbl)
                n407 = Add(x=w437, y=w443) -> (x+y=w439:dbl)
                n408 = Add(x=w436, y=w442) -> (x+y=w438:dbl)
                n409 = Less Or Equal?(x=w439, y=0) -> (x <= y?=w445:bool)
                n410 = Greater Or Equal?(x=w438, y=w441) -> (x >= y?=w444:bool)
                n411 = property on="P5" class="Bool (strict)"("Left"=w439, "Top"=w438) -> ()  [unwired: 2 in, 2 out]
                n412 = case shown="True" w445 {
                  tunnel: w444 -> [w446 w448]
                  frame False {
                    n413 = case shown="False" w446 {
                      frame False {
                      }
                      frame True {
                        n414 = local write "State 5"(T1."Left-up" ("State")) -> ()
                      }
                    }
                  }
                  frame True {
                    n415 = case shown="True" w448 {
                      frame False {
                        n416 = local write "State 5"(T1."Right-down" ("State")) -> ()
                      }
                      frame True {
                        n417 = local write "State 5"(T1."Right-up" ("State")) -> ()
                      }
                    }
                  }
                }
              }
              frame "Right-down", Default {
                n418 = call "Plus&Stay.vi"() -> ("s? t:f"=w451:dbl)
                n419 = call "Plus&Stay.vi"() -> ("s? t:f"=w453:dbl)
                n420 = local read "Bound bottom"() -> (w458:dbl)
                n421 = local read "Bound right"() -> (w459:dbl)
                n422 = Add(x=w453, y=w460) -> (x+y=w455:dbl)
                n423 = Add(x=w452, y=w451) -> (x+y=w454:dbl)
                n424 = Greater Or Equal?(x=w455, y=w459) -> (x >= y?=w457:bool)
                n425 = Greater Or Equal?(x=w454, y=w458) -> (x >= y?=w456:bool)
                n426 = property on="P5" class="Bool (strict)"("Left"=w455, "Top"=w454) -> ()  [unwired: 2 in, 2 out]
                n427 = case shown="True" w457 {
                  tunnel: w456 -> [w461 w463]
                  frame False {
                    n428 = case shown="False" w461 {
                      frame False {
                      }
                      frame True {
                        n429 = local write "State 5"(T1."Right-up" ("State")) -> ()
                      }
                    }
                  }
                  frame True {
                    n430 = case shown="False" w463 {
                      frame False {
                        n431 = local write "State 5"(T1."Left-down" ("State")) -> ()
                      }
                      frame True {
                        n432 = local write "State 5"(T1."Left-up" ("State")) -> ()
                      }
                    }
                  }
                }
              }
              frame "Left-up" {
                w471 = 0 ("y")
                n433 = call "Minus&Stay.vi"() -> ("s? t:f"=w468:dbl)
                n434 = call "Minus&Stay.vi"() -> ("s? t:f"=w466:dbl)
                n435 = Add(x=w468, y=w472) -> (x+y=w470:dbl)
                n436 = Add(x=w467, y=w466) -> (x+y=w469:dbl)
                n437 = Less Or Equal?(x=w470, y=w471) -> (x <= y?=w474:bool)
                n438 = Less Or Equal?(x=w469, y=w471) -> (x <= y?=w473:bool)
                n439 = property on="P5" class="Bool (strict)"("Left"=w470, "Top"=w469) -> ()  [unwired: 2 in, 2 out]
                n440 = case shown="False" w474 {
                  tunnel: w473 -> [w475 w477]
                  frame False {
                    n441 = case shown="True" w475 {
                      frame False {
                      }
                      frame True {
                        n442 = local write "State 5"(T1."Left-down" ("State")) -> ()
                      }
                    }
                  }
                  frame True {
                    n443 = case shown="True" w477 {
                      frame False {
                        n444 = local write "State 5"(T1."Right-up" ("State")) -> ()
                      }
                      frame True {
                        n445 = local write "State 5"(T1."Right-down" ("State")) -> ()
                      }
                    }
                  }
                }
              }
            }
            n446 = case shown="\"Right-down\", Default" w125 {
              tunnel: w124 -> [w661 w677 w696 w706]
              tunnel: w123 -> [w658 w673 w688 w703]
              frame "Right-up" {
                n447 = call "Minus&Stay.vi"() -> ("s? t:f"=w657:dbl)
                n448 = call "Plus&Stay.vi"() -> ("s? t:f"=w659:dbl)
                n449 = Add(x=w659, y=w661) -> (x+y=w665:dbl)
                n450 = Add(x=w658, y=w657) -> (x+y=w664:dbl)
                n451 = local read "Bound right"() -> (w666:dbl)
                n452 = Greater Or Equal?(x=w665, y=w666) -> (x >= y?=w663:bool)
                n453 = Less Or Equal?(x=w664, y=0) -> (x <= y?=w662:bool)
                n454 = property on="P1" class="Bool (strict)"("Left"=w665, "Top"=w664) -> ()  [unwired: 2 in, 2 out]
                n455 = case shown="False" w663 {
                  tunnel: w662 -> [w667 w669]
                  frame False {
                    n456 = case shown="False" w667 {
                      frame False {
                      }
                      frame True {
                        n457 = local write "State"(T1."Right-down" ("State")) -> ()
                      }
                    }
                  }
                  frame True {
                    n458 = case shown="False" w669 {
                      frame False {
                        n459 = local write "State"(T1."Left-up" ("State")) -> ()
                      }
                      frame True {
                        n460 = local write "State"(T1."Left-down" ("State")) -> ()
                      }
                    }
                  }
                }
              }
              frame "Left-down" {
                n461 = call "Plus&Stay.vi"() -> ("s? t:f"=w672:dbl)
                n462 = call "Minus&Stay.vi"() -> ("s? t:f"=w674:dbl)
                n463 = Add(x=w674, y=w677) -> (x+y=w681:dbl)
                n464 = local read "Bound bottom"() -> (w676:dbl)
                n465 = Add(x=w673, y=w672) -> (x+y=w680:dbl)
                n466 = Less Or Equal?(x=w681, y=0) -> (x <= y?=w679:bool)
                n467 = Greater Or Equal?(x=w680, y=w676) -> (x >= y?=w678:bool)
                n468 = property on="P1" class="Bool (strict)"("Left"=w681, "Top"=w680) -> ()  [unwired: 2 in, 2 out]
                n469 = case shown="False" w679 {
                  tunnel: w678 -> [w682 w684]
                  frame False {
                    n470 = case shown="True" w682 {
                      frame False {
                      }
                      frame True {
                        n471 = local write "State"(T1."Left-up" ("State")) -> ()
                      }
                    }
                  }
                  frame True {
                    n472 = case shown="False" w684 {
                      frame False {
                        n473 = local write "State"(T1."Right-down" ("State")) -> ()
                      }
                      frame True {
                        n474 = local write "State"(T1."Right-up" ("State")) -> ()
                      }
                    }
                  }
                }
              }
              frame "Right-down", Default {
                n475 = local read "Bound bottom"() -> (w694:dbl)
                n476 = call "Plus&Stay.vi"() -> ("s? t:f"=w687:dbl)
                n477 = call "Plus&Stay.vi"() -> ("s? t:f"=w689:dbl)
                n478 = local read "Bound right"() -> (w695:dbl)
                n479 = Add(x=w688, y=w687) -> (x+y=w690:dbl)
                n480 = Add(x=w689, y=w696) -> (x+y=w693:dbl)
                n481 = Greater Or Equal?(x=w693, y=w695) -> (x >= y?=w692:bool)
                n482 = Greater Or Equal?(x=w690, y=w694) -> (x >= y?=w691:bool)
                n483 = property on="P1" class="Bool (strict)"("Left"=w693, "Top"=w690) -> ()  [unwired: 2 in, 2 out]
                n484 = case shown="False" w692 {
                  tunnel: w691 -> [w697 w699]
                  frame False {
                    n485 = case shown="False" w697 {
                      frame False {
                      }
                      frame True {
                        n486 = local write "State"(T1."Right-up" ("State")) -> ()
                      }
                    }
                  }
                  frame True {
                    n487 = case shown="False" w699 {
                      frame False {
                        n488 = local write "State"(T1."Left-down" ("State")) -> ()
                      }
                      frame True {
                        n489 = local write "State"(T1."Left-up" ("State")) -> ()
                      }
                    }
                  }
                }
              }
              frame "Left-up" {
                w705 = 0 ("y")
                n490 = call "Minus&Stay.vi"() -> ("s? t:f"=w702:dbl)
                n491 = call "Minus&Stay.vi"() -> ("s? t:f"=w704:dbl)
                n492 = Add(x=w704, y=w706) -> (x+y=w710:dbl)
                n493 = Add(x=w703, y=w702) -> (x+y=w709:dbl)
                n494 = Less Or Equal?(x=w710, y=w705) -> (x <= y?=w708:bool)
                n495 = Less Or Equal?(x=w709, y=w705) -> (x <= y?=w707:bool)
                n496 = property on="P1" class="Bool (strict)"("Left"=w710, "Top"=w709) -> ()  [unwired: 2 in, 2 out]
                n497 = case shown="False" w708 {
                  tunnel: w707 -> [w711 w713]
                  frame False {
                    n498 = case shown="True" w711 {
                      frame False {
                      }
                      frame True {
                        n499 = local write "State"(T1."Left-down" ("State")) -> ()
                      }
                    }
                  }
                  frame True {
                    n500 = case shown="False" w713 {
                      frame False {
                        n501 = local write "State"(T1."Right-up" ("State")) -> ()
                      }
                      frame True {
                        n502 = local write "State"(T1."Right-down" ("State")) -> ()
                      }
                    }
                  }
                }
              }
            }
            n503 = case shown="\"Right-up\"" w105 {
              tunnel: w104 -> [w309 w325 w342 w354]
              tunnel: w106 -> [w308 w324 w334 w349]
              frame "Right-up" {
                n504 = call "Minus&Stay.vi"() -> ("s? t:f"=w303:dbl)
                n505 = call "Plus&Stay.vi"() -> ("s? t:f"=w304:dbl)
                n506 = Add(x=w304, y=w309) -> (x+y=w306:dbl)
                n507 = Add(x=w303, y=w308) -> (x+y=w305:dbl)
                n508 = local read "Bound right"() -> (w312:dbl)
                n509 = Greater Or Equal?(x=w306, y=w312) -> (x >= y?=w311:bool)
                n510 = Less Or Equal?(x=w305, y=0) -> (x <= y?=w310:bool)
                n511 = property on="P7" class="Bool (strict)"("Left"=w306, "Top"=w305) -> ()  [unwired: 2 in, 2 out]
                n512 = case shown="True" w311 {
                  tunnel: w310 -> [w313 w315]
                  frame False {
                    n513 = case shown="True" w313 {
                      frame False {
                      }
                      frame True {
                        n514 = local write "State 7"(T1."Right-down" ("State")) -> ()
                      }
                    }
                  }
                  frame True {
                    n515 = case shown="True" w315 {
                      frame False {
                        n516 = local write "State 7"(T1."Left-up" ("State")) -> ()
                      }
                      frame True {
                        n517 = local write "State 7"(T1."Left-down" ("State")) -> ()
                      }
                    }
                  }
                }
              }
              frame "Left-down" {
                n518 = call "Plus&Stay.vi"() -> ("s? t:f"=w318:dbl)
                n519 = call "Minus&Stay.vi"() -> ("s? t:f"=w319:dbl)
                n520 = local read "Bound bottom"() -> (w323:dbl)
                n521 = Add(x=w319, y=w325) -> (x+y=w321:dbl)
                n522 = Add(x=w318, y=w324) -> (x+y=w320:dbl)
                n523 = Less Or Equal?(x=w321, y=0) -> (x <= y?=w327:bool)
                n524 = Greater Or Equal?(x=w320, y=w323) -> (x >= y?=w326:bool)
                n525 = property on="P7" class="Bool (strict)"("Left"=w321, "Top"=w320) -> ()  [unwired: 2 in, 2 out]
                n526 = case shown="True" w327 {
                  tunnel: w326 -> [w328 w330]
                  frame False {
                    n527 = case shown="True" w328 {
                      frame False {
                      }
                      frame True {
                        n528 = local write "State 7"(T1."Left-up" ("State")) -> ()
                      }
                    }
                  }
                  frame True {
                    n529 = case shown="True" w330 {
                      frame False {
                        n530 = local write "State 7"(T1."Right-down" ("State")) -> ()
                      }
                      frame True {
                        n531 = local write "State 7"(T1."Right-up" ("State")) -> ()
                      }
                    }
                  }
                }
              }
              frame "Right-down", Default {
                n532 = call "Plus&Stay.vi"() -> ("s? t:f"=w333:dbl)
                n533 = call "Plus&Stay.vi"() -> ("s? t:f"=w335:dbl)
                n534 = local read "Bound bottom"() -> (w340:dbl)
                n535 = local read "Bound right"() -> (w341:dbl)
                n536 = Add(x=w335, y=w342) -> (x+y=w337:dbl)
                n537 = Add(x=w334, y=w333) -> (x+y=w336:dbl)
                n538 = Greater Or Equal?(x=w337, y=w341) -> (x >= y?=w339:bool)
                n539 = Greater Or Equal?(x=w336, y=w340) -> (x >= y?=w338:bool)
                n540 = property on="P7" class="Bool (strict)"("Left"=w337, "Top"=w336) -> ()  [unwired: 2 in, 2 out]
                n541 = case shown="True" w339 {
                  tunnel: w338 -> [w343 w345]
                  frame False {
                    n542 = case shown="True" w343 {
                      frame False {
                      }
                      frame True {
                        n543 = local write "State 7"(T1."Right-up" ("State")) -> ()
                      }
                    }
                  }
                  frame True {
                    n544 = case shown="False" w345 {
                      frame False {
                        n545 = local write "State 7"(T1."Left-down" ("State")) -> ()
                      }
                      frame True {
                        n546 = local write "State 7"(T1."Left-up" ("State")) -> ()
                      }
                    }
                  }
                }
              }
              frame "Left-up" {
                w353 = 0 ("y")
                n547 = call "Minus&Stay.vi"() -> ("s? t:f"=w350:dbl)
                n548 = call "Minus&Stay.vi"() -> ("s? t:f"=w348:dbl)
                n549 = Add(x=w350, y=w354) -> (x+y=w352:dbl)
                n550 = Add(x=w349, y=w348) -> (x+y=w351:dbl)
                n551 = Less Or Equal?(x=w352, y=w353) -> (x <= y?=w356:bool)
                n552 = Less Or Equal?(x=w351, y=w353) -> (x <= y?=w355:bool)
                n553 = property on="P7" class="Bool (strict)"("Left"=w352, "Top"=w351) -> ()  [unwired: 2 in, 2 out]
                n554 = case shown="False" w356 {
                  tunnel: w355 -> [w357 w359]
                  frame False {
                    n555 = case shown="True" w357 {
                      frame False {
                      }
                      frame True {
                        n556 = local write "State 7"(T1."Left-down" ("State")) -> ()
                      }
                    }
                  }
                  frame True {
                    n557 = case shown="True" w359 {
                      frame False {
                        n558 = local write "State 7"(T1."Right-up" ("State")) -> ()
                      }
                      frame True {
                        n559 = local write "State 7"(T1."Right-down" ("State")) -> ()
                      }
                    }
                  }
                }
              }
            }
            n560 = case shown="\"Left-up\"" w102 {
              tunnel: w103 -> [w250 w266 w283 w295]
              tunnel: w101 -> [w249 w265 w275 w290]
              frame "Right-up" {
                n561 = call "Minus&Stay.vi"() -> ("s? t:f"=w244:dbl)
                n562 = call "Plus&Stay.vi"() -> ("s? t:f"=w245:dbl)
                n563 = Add(x=w245, y=w250) -> (x+y=w247:dbl)
                n564 = Add(x=w244, y=w249) -> (x+y=w246:dbl)
                n565 = local read "Bound right"() -> (w253:dbl)
                n566 = Greater Or Equal?(x=w247, y=w253) -> (x >= y?=w252:bool)
                n567 = Less Or Equal?(x=w246, y=0) -> (x <= y?=w251:bool)
                n568 = property on="P8" class="Bool (strict)"("Left"=w247, "Top"=w246) -> ()  [unwired: 2 in, 2 out]
                n569 = case shown="False" w252 {
                  tunnel: w251 -> [w254 w256]
                  frame False {
                    n570 = case shown="True" w254 {
                      frame False {
                      }
                      frame True {
                        n571 = local write "State 8"(T1."Right-down" ("State")) -> ()
                      }
                    }
                  }
                  frame True {
                    n572 = case shown="False" w256 {
                      frame False {
                        n573 = local write "State 8"(T1."Left-up" ("State")) -> ()
                      }
                      frame True {
                        n574 = local write "State 8"(T1."Left-down" ("State")) -> ()
                      }
                    }
                  }
                }
              }
              frame "Left-down" {
                n575 = call "Plus&Stay.vi"() -> ("s? t:f"=w259:dbl)
                n576 = call "Minus&Stay.vi"() -> ("s? t:f"=w260:dbl)
                n577 = local read "Bound bottom"() -> (w264:dbl)
                n578 = Add(x=w260, y=w266) -> (x+y=w262:dbl)
                n579 = Add(x=w259, y=w265) -> (x+y=w261:dbl)
                n580 = Less Or Equal?(x=w262, y=0) -> (x <= y?=w268:bool)
                n581 = Greater Or Equal?(x=w261, y=w264) -> (x >= y?=w267:bool)
                n582 = property on="P8" class="Bool (strict)"("Left"=w262, "Top"=w261) -> ()  [unwired: 2 in, 2 out]
                n583 = case shown="False" w268 {
                  tunnel: w267 -> [w269 w271]
                  frame False {
                    n584 = case shown="True" w269 {
                      frame False {
                      }
                      frame True {
                        n585 = local write "State 8"(T1."Left-up" ("State")) -> ()
                      }
                    }
                  }
                  frame True {
                    n586 = case shown="False" w271 {
                      frame False {
                        n587 = local write "State 8"(T1."Right-down" ("State")) -> ()
                      }
                      frame True {
                        n588 = local write "State 8"(T1."Right-up" ("State")) -> ()
                      }
                    }
                  }
                }
              }
              frame "Right-down", Default {
                n589 = call "Plus&Stay.vi"() -> ("s? t:f"=w274:dbl)
                n590 = call "Plus&Stay.vi"() -> ("s? t:f"=w276:dbl)
                n591 = local read "Bound bottom"() -> (w281:dbl)
                n592 = local read "Bound right"() -> (w282:dbl)
                n593 = Add(x=w276, y=w283) -> (x+y=w278:dbl)
                n594 = Add(x=w275, y=w274) -> (x+y=w277:dbl)
                n595 = Greater Or Equal?(x=w278, y=w282) -> (x >= y?=w280:bool)
                n596 = Greater Or Equal?(x=w277, y=w281) -> (x >= y?=w279:bool)
                n597 = property on="P8" class="Bool (strict)"("Left"=w278, "Top"=w277) -> ()  [unwired: 2 in, 2 out]
                n598 = case shown="False" w280 {
                  tunnel: w279 -> [w284 w286]
                  frame False {
                    n599 = case shown="True" w284 {
                      frame False {
                      }
                      frame True {
                        n600 = local write "State 8"(T1."Right-up" ("State")) -> ()
                      }
                    }
                  }
                  frame True {
                    n601 = case shown="True" w286 {
                      frame False {
                        n602 = local write "State 8"(T1."Left-down" ("State")) -> ()
                      }
                      frame True {
                        n603 = local write "State 8"(T1."Left-up" ("State")) -> ()
                      }
                    }
                  }
                }
              }
              frame "Left-up" {
                w294 = 0 ("y")
                n604 = call "Minus&Stay.vi"() -> ("s? t:f"=w291:dbl)
                n605 = call "Minus&Stay.vi"() -> ("s? t:f"=w289:dbl)
                n606 = Add(x=w291, y=w295) -> (x+y=w293:dbl)
                n607 = Add(x=w290, y=w289) -> (x+y=w292:dbl)
                n608 = Less Or Equal?(x=w293, y=w294) -> (x <= y?=w297:bool)
                n609 = Less Or Equal?(x=w292, y=w294) -> (x <= y?=w296:bool)
                n610 = property on="P8" class="Bool (strict)"("Left"=w293, "Top"=w292) -> ()  [unwired: 2 in, 2 out]
                n611 = case shown="False" w297 {
                  tunnel: w296 -> [w298 w300]
                  frame False {
                    n612 = case shown="False" w298 {
                      frame False {
                      }
                      frame True {
                        n613 = local write "State 8"(T1."Left-down" ("State")) -> ()
                      }
                    }
                  }
                  frame True {
                    n614 = case shown="False" w300 {
                      frame False {
                        n615 = local write "State 8"(T1."Right-up" ("State")) -> ()
                      }
                      frame True {
                        n616 = local write "State 8"(T1."Right-down" ("State")) -> ()
                      }
                    }
                  }
                }
              }
            }
          }
          frame #1 {
            w770 = 0 ("x")
            w719 = 250 ("y")
            n617 = property on="P4" class="Bool (strict)"() -> ("Left"=w746:i32)  [unwired: 2 in, 2 out]
            n618 = property on="P5" class="Bool (strict)"() -> ("Left"=w743:i32)  [unwired: 2 in, 2 out]
            n619 = property on="P1" class="Bool (strict)"() -> ("Left"=w747:i32)  [unwired: 2 in, 2 out]
            n620 = property on="P2" class="Bool (strict)"() -> ("Left"=w748:i32)  [unwired: 2 in, 2 out]
            n621 = property on="P3" class="Bool (strict)"() -> ("Left"=w755:i32)  [unwired: 2 in, 2 out]
            n622 = property on="P6" class="Bool (strict)"() -> ("Left"=w740:i32)  [unwired: 2 in, 2 out]
            n623 = property on="P7" class="Bool (strict)"() -> ("Left"=w737:i32)  [unwired: 2 in, 2 out]
            n624 = property on="P8" class="Bool (strict)"() -> ("Left"=w734:i32)  [unwired: 2 in, 2 out]
            n625 = property on="P9" class="Bool (strict)"() -> ("Left"=w731:i32)  [unwired: 2 in, 2 out]
            n626 = property on="P10" class="Bool (strict)"() -> ("Left"=w728:i32)  [unwired: 2 in, 2 out]
            n627 = property on="P6" class="Bool (strict)"() -> ("Top"=w739:i32)  [unwired: 2 in, 2 out]
            n628 = property on="P7" class="Bool (strict)"() -> ("Top"=w736:i32)  [unwired: 2 in, 2 out]
            n629 = property on="P5" class="Bool (strict)"() -> ("Value"=w741:bool)  [unwired: 2 in, 2 out]
            n630 = property on="P1" class="Bool (strict)"() -> ("Value"=w751:bool)  [unwired: 2 in, 2 out]
            n631 = property on="P2" class="Bool (strict)"() -> ("Value"=w752:bool)  [unwired: 2 in, 2 out]
            n632 = property on="P3" class="Bool (strict)"() -> ("Value"=w753:bool)  [unwired: 2 in, 2 out]
            n633 = property on="P4" class="Bool (strict)"() -> ("Value"=w744:bool)  [unwired: 2 in, 2 out]
            n634 = property on="P6" class="Bool (strict)"() -> ("Value"=w738:bool)  [unwired: 2 in, 2 out]
            n635 = property on="P9" class="Bool (strict)"() -> ("Top"=w730:i32)  [unwired: 2 in, 2 out]
            n636 = property on="P10" class="Bool (strict)"() -> ("Top"=w727:i32)  [unwired: 2 in, 2 out]
            n637 = property on="P8" class="Bool (strict)"() -> ("Top"=w733:i32)  [unwired: 2 in, 2 out]
            n638 = property on="P7" class="Bool (strict)"() -> ("Value"=w735:bool)  [unwired: 2 in, 2 out]
            n639 = property on="P1" class="Bool (strict)"() -> ("Top"=w750:i32)  [unwired: 2 in, 2 out]
            n640 = property on="P2" class="Bool (strict)"() -> ("Top"=w749:i32)  [unwired: 2 in, 2 out]
            n641 = property on="P3" class="Bool (strict)"() -> ("Top"=w754:i32)  [unwired: 2 in, 2 out]
            n642 = property on="P4" class="Bool (strict)"() -> ("Top"=w745:i32)  [unwired: 2 in, 2 out]
            n643 = property on="P5" class="Bool (strict)"() -> ("Top"=w742:i32)  [unwired: 2 in, 2 out]
            n644 = property on="P8" class="Bool (strict)"() -> ("Value"=w732:bool)  [unwired: 2 in, 2 out]
            n645 = property on="P9" class="Bool (strict)"() -> ("Value"=w729:bool)  [unwired: 2 in, 2 out]
            n646 = property on="P10" class="Bool (strict)"() -> ("Value"=w726:bool)  [unwired: 2 in, 2 out]
            n647 = Build Array(w747, w748, w755, w746, w743, w740, w737, w734, w731, w728) -> (w764:i32[])
            "X" <- w764
            n648 = Build Array(w750, w749, w754, w745, w742, w739, w736, w733, w730, w727) -> (w763:i32[])
            "Y" <- w763
            n649 = Build Array(w751, w752, w753, w744, w741, w738, w735, w732, w729, w726) -> (w762:bool[])
            n650 = Divide(x="再感染機率", y=100.0) -> (x/y=w716:dbl)
            n651 = Random Number (0-1)() -> (number: 0 to 1=w724:dbl)
            n652 = Less Or Equal?(x=w724, y=w716) -> (x <= y?=w723:bool)
            n653 = Greater Or Equal?(x=w719, y=w720) -> (x >= y?=w722:bool)
            n654 = Quotient & Remainder(x=w720, y=w719) -> (x-y*floor(x/y)=w771:i32)  [unwired: 1 out]
            n655 = call "DistanceStatus.vi"("Status i"=w762, "Y"=w763, "X"=w764) -> ("Status i+1"=w768:bool[])
            n656 = Not Equal?(x=w720, y=w770) -> (x != y?=w769:bool)
            n657 = Or(x=w722, y=w723) -> (x .or. y?=w721:bool)
            n658 = Equal?(x=w770, y=w771) -> (x = y?=w766:bool)
            n659 = Divide(x="陰轉陽率", y=100.0) -> (x/y=w759:dbl)
            n660 = And(x=w769, y=w766) -> (x .and. y?=w767:bool)
            n661 = case shown="False" w767 {
              tunnel: w761 -> [_ w1003]
              tunnel: [w825 w1030] -> w760
              tunnel: w768 -> [w776 w1004]
              tunnel: w759 -> [_ w970]
              tunnel: "死亡率" -> [_ w969]
              tunnel: cluster{u32, u32}[] [{16860, 16860}] ("Colors [4]") -> [_ w967]
              tunnel: w721 -> [w774 _]
              frame False {
                n662 = local read "P2 Infeted?"() -> (w820:enum16{"Infected", "Uninfected"})
                n663 = local read "P3 Infeted?"() -> (w812:enum16{"Infected", "Uninfected"})
                n664 = local read "P4 Infeted?"() -> (w810:enum16{"Infected", "Uninfected"})
                n665 = local read "P5 Infeted?"() -> (w803:enum16{"Infected", "Uninfected"})
                n666 = local read "P6 Infeted?"() -> (w800:enum16{"Infected", "Uninfected"})
                n667 = local read "P10 Infeted"() -> (w780:enum16{"Infected", "Uninfected"})
                n668 = local read "P1 Infeted?"() -> (w821:enum16{"Infected", "Uninfected"})
                n669 = local read "P7 Infeted?"() -> (w792:enum16{"Infected", "Uninfected"})
                n670 = local read "P8 Infeted?"() -> (w790:enum16{"Infected", "Uninfected"})
                n671 = local read "P9 Infeted?"() -> (w782:enum16{"Infected", "Uninfected"})
                n672 = Index Array(array=w776, index=1) -> (element=w819:bool)
                n673 = Index Array(array=w776, index=2) -> (element=w813:bool)
                n674 = Index Array(array=w776, index=3) -> (element=w809:bool)
                n675 = Index Array(array=w776, index=4) -> (element=w804:bool)
                n676 = Index Array(array=w776, index=5) -> (element=w799:bool)
                n677 = Index Array(array=w776, index=0) -> (element=w822:bool)
                n678 = Index Array(array=w776, index=6) -> (element=w793:bool)
                n679 = Index Array(array=w776, index=7) -> (element=w789:bool)
                n680 = Index Array(array=w776, index=8) -> (element=w783:bool)
                n681 = Index Array(array=w776, index=9) -> (element=w779:bool)
                n682 = local read "Alive? P10"() -> (w777:enum16{"Alive", "Dead"})
                n683 = local read "Alive? P2"() -> (w817:enum16{"Alive", "Dead"})
                n684 = local read "Alive? P3"() -> (w815:enum16{"Alive", "Dead"})
                n685 = local read "Alive? P4"() -> (w807:enum16{"Alive", "Dead"})
                n686 = local read "Alive? P5"() -> (w806:enum16{"Alive", "Dead"})
                n687 = local read "Alive? P6"() -> (w797:enum16{"Alive", "Dead"})
                n688 = local read "Alive? P1"() -> (w824:enum16{"Alive", "Dead"})
                n689 = local read "Alive? P7"() -> (w795:enum16{"Alive", "Dead"})
                n690 = local read "Alive? P8"() -> (w787:enum16{"Alive", "Dead"})
                n691 = local read "Alive? P9"() -> (w785:enum16{"Alive", "Dead"})
                n692 = case shown="\"Alive\", Default" w817 {
                  tunnel: w819 -> [w942 _]
                  tunnel: [w941 w952] -> w816
                  tunnel: w820 -> [w940 _]
                  tunnel: w774 -> [w939 _]
                  frame "Alive", Default {
                    n693 = case shown="\"Uninfected\"" w940 {
                      tunnel: w942 -> [w945 w951]
                      tunnel: [w944 w951] -> w941
                      tunnel: w939 -> [w943 _]
                      frame "Infected", Default {
                        n694 = case shown="False" w945 {
                          selector: w945 -> [w946 w950]
                          tunnel: [w946 w948] -> w944
                          tunnel: w943 -> [_ w947]
                          frame False {
                            n695 = local write "P2"(w946) -> ()
                          }
                          frame True {
                            n696 = Select(t=w950, s=w947, f=FALSE) -> (s? t:f=w948:bool)
                            n697 = local write "P2"(w948) -> ()
                          }
                        }
                      }
                      frame "Uninfected" {
                        n698 = local write "P2"(w951) -> ()
                      }
                    }
                  }
                  frame "Dead" {
                    w952 = FALSE ("P1")
                    n699 = local write "P2"(w952) -> ()
                  }
                }
                n700 = case shown="\"Alive\", Default" w815 {
                  tunnel: w813 -> [w928 _]
                  tunnel: [w927 w938] -> w811
                  tunnel: w812 -> [w926 _]
                  tunnel: w774 -> [w925 _]
                  frame "Alive", Default {
                    n701 = case shown="\"Uninfected\"" w926 {
                      tunnel: w928 -> [w931 w937]
                      tunnel: [w930 w937] -> w927
                      tunnel: w925 -> [w929 _]
                      frame "Infected", Default {
                        n702 = case shown="False" w931 {
                          selector: w931 -> [w932 w936]
                          tunnel: [w932 w934] -> w930
                          tunnel: w929 -> [_ w933]
                          frame False {
                            n703 = local write "P3"(w932) -> ()
                          }
                          frame True {
                            n704 = Select(t=w936, s=w933, f=FALSE) -> (s? t:f=w934:bool)
                            n705 = local write "P3"(w934) -> ()
                          }
                        }
                      }
                      frame "Uninfected" {
                        n706 = local write "P3"(w937) -> ()
                      }
                    }
                  }
                  frame "Dead" {
                    w938 = FALSE ("P1")
                    n707 = local write "P3"(w938) -> ()
                  }
                }
                n708 = case shown="\"Alive\", Default" w807 {
                  tunnel: w809 -> [w914 _]
                  tunnel: [w913 w924] -> w802
                  tunnel: w810 -> [w912 _]
                  tunnel: w774 -> [w911 _]
                  frame "Alive", Default {
                    n709 = case shown="\"Uninfected\"" w912 {
                      tunnel: w914 -> [w917 w923]
                      tunnel: [w916 w923] -> w913
                      tunnel: w911 -> [w915 _]
                      frame "Infected", Default {
                        n710 = case shown="True" w917 {
                          selector: w917 -> [w918 w922]
                          tunnel: [w918 w920] -> w916
                          tunnel: w915 -> [_ w919]
                          frame False {
                            n711 = local write "P4"(w918) -> ()
                          }
                          frame True {
                            n712 = Select(t=w922, s=w919, f=FALSE) -> (s? t:f=w920:bool)
                            n713 = local write "P4"(w920) -> ()
                          }
                        }
                      }
                      frame "Uninfected" {
                        n714 = local write "P4"(w923) -> ()
                      }
                    }
                  }
                  frame "Dead" {
                    w924 = FALSE ("P1")
                    n715 = local write "P4"(w924) -> ()
                  }
                }
                n716 = case shown="\"Alive\", Default" w806 {
                  tunnel: w804 -> [w900 _]
                  tunnel: [w899 w910] -> w801
                  tunnel: w803 -> [w898 _]
                  tunnel: w774 -> [w897 _]
                  frame "Alive", Default {
                    n717 = case shown="\"Infected\", Default" w898 {
                      tunnel: w900 -> [w903 w909]
                      tunnel: [w902 w909] -> w899
                      tunnel: w897 -> [w901 _]
                      frame "Infected", Default {
                        n718 = case shown="True" w903 {
                          selector: w903 -> [w904 w908]
                          tunnel: [w904 w906] -> w902
                          tunnel: w901 -> [_ w905]
                          frame False {
                            n719 = local write "P5"(w904) -> ()
                          }
                          frame True {
                            n720 = Select(t=w908, s=w905, f=FALSE) -> (s? t:f=w906:bool)
                            n721 = local write "P5"(w906) -> ()
                          }
                        }
                      }
                      frame "Uninfected" {
                        n722 = local write "P5"(w909) -> ()
                      }
                    }
                  }
                  frame "Dead" {
                    w910 = FALSE ("P1")
                    n723 = local write "P5"(w910) -> ()
                  }
                }
                n724 = case shown="\"Alive\", Default" w797 {
                  tunnel: w799 -> [w886 _]
                  tunnel: [w885 w896] -> w796
                  tunnel: w800 -> [w884 _]
                  tunnel: w774 -> [w883 _]
                  frame "Alive", Default {
                    n725 = case shown="\"Uninfected\"" w884 {
                      tunnel: w886 -> [w889 w895]
                      tunnel: [w888 w895] -> w885
                      tunnel: w883 -> [w887 _]
                      frame "Infected", Default {
                        n726 = case shown="False" w889 {
                          selector: w889 -> [w890 w894]
                          tunnel: [w890 w892] -> w888
                          tunnel: w887 -> [_ w891]
                          frame False {
                            n727 = local write "P6"(w890) -> ()
                          }
                          frame True {
                            n728 = Select(t=w894, s=w891, f=FALSE) -> (s? t:f=w892:bool)
                            n729 = local write "P6"(w892) -> ()
                          }
                        }
                      }
                      frame "Uninfected" {
                        n730 = local write "P6"(w895) -> ()
                      }
                    }
                  }
                  frame "Dead" {
                    w896 = FALSE ("P1")
                    n731 = local write "P6"(w896) -> ()
                  }
                }
                n732 = case shown="\"Alive\", Default" w824 {
                  tunnel: w822 -> [w956 _]
                  tunnel: [w955 w966] -> w826
                  tunnel: w821 -> [w954 _]
                  tunnel: w774 -> [w953 _]
                  frame "Alive", Default {
                    n733 = case shown="\"Uninfected\"" w954 {
                      tunnel: w956 -> [w959 w965]
                      tunnel: [w958 w965] -> w955
                      tunnel: w953 -> [w957 _]
                      frame "Infected", Default {
                        n734 = case shown="True" w959 {
                          selector: w959 -> [w960 w964]
                          tunnel: [w960 w962] -> w958
                          tunnel: w957 -> [_ w961]
                          frame False {
                            # "維持當下狀態"
                            n735 = local write "P1"(w960) -> ()
                          }
                          frame True {
                            # "已經染疫過，\n機率決定是否再染疫"
                            n736 = Select(t=w964, s=w961, f=FALSE) -> (s? t:f=w962:bool)
                            n737 = local write "P1"(w962) -> ()
                          }
                        }
                      }
                      frame "Uninfected" {
                        # "若未染疫過只要出現過TRUE便會在這個\nCASE內使狀態轉為Infected"
                        n738 = local write "P1"(w965) -> ()
                      }
                    }
                  }
                  frame "Dead" {
                    w966 = FALSE ("P1")
                    # "已死亡輸出為False"
                    n739 = local write "P1"(w966) -> ()
                  }
                }
                n740 = case shown="\"Alive\", Default" w795 {
                  tunnel: w793 -> [w872 _]
                  tunnel: [w871 w882] -> w791
                  tunnel: w792 -> [w870 _]
                  tunnel: w774 -> [w869 _]
                  frame "Alive", Default {
                    n741 = case shown="\"Uninfected\"" w870 {
                      tunnel: w872 -> [w875 w881]
                      tunnel: [w874 w881] -> w871
                      tunnel: w869 -> [w873 _]
                      frame "Infected", Default {
                        n742 = case shown="False" w875 {
                          selector: w875 -> [w876 w880]
                          tunnel: [w876 w878] -> w874
                          tunnel: w873 -> [_ w877]
                          frame False {
                            n743 = local write "P7"(w876) -> ()
                          }
                          frame True {
                            n744 = Select(t=w880, s=w877, f=FALSE) -> (s? t:f=w878:bool)
                            n745 = local write "P7"(w878) -> ()
                          }
                        }
                      }
                      frame "Uninfected" {
                        n746 = local write "P7"(w881) -> ()
                      }
                    }
                  }
                  frame "Dead" {
                    w882 = FALSE ("P1")
                    n747 = local write "P7"(w882) -> ()
                  }
                }
                n748 = case shown="\"Alive\", Default" w787 {
                  tunnel: w789 -> [w858 _]
                  tunnel: [w857 w868] -> w786
                  tunnel: w790 -> [w856 _]
                  tunnel: w774 -> [w855 _]
                  frame "Alive", Default {
                    n749 = case shown="\"Uninfected\"" w856 {
                      tunnel: w858 -> [w861 w867]
                      tunnel: [w860 w867] -> w857
                      tunnel: w855 -> [w859 _]
                      frame "Infected", Default {
                        n750 = case shown="True" w861 {
                          selector: w861 -> [w862 w866]
                          tunnel: [w862 w864] -> w860
                          tunnel: w859 -> [_ w863]
                          frame False {
                            n751 = local write "P8"(w862) -> ()
                          }
                          frame True {
                            n752 = Select(t=w866, s=w863, f=FALSE) -> (s? t:f=w864:bool)
                            n753 = local write "P8"(w864) -> ()
                          }
                        }
                      }
                      frame "Uninfected" {
                        n754 = local write "P8"(w867) -> ()
                      }
                    }
                  }
                  frame "Dead" {
                    w868 = FALSE ("P1")
                    n755 = local write "P8"(w868) -> ()
                  }
                }
                n756 = case shown="\"Alive\", Default" w785 {
                  tunnel: w783 -> [w844 _]
                  tunnel: [w843 w854] -> w781
                  tunnel: w782 -> [w842 _]
                  tunnel: w774 -> [w841 _]
                  frame "Alive", Default {
                    n757 = case shown="\"Uninfected\"" w842 {
                      tunnel: w844 -> [w847 w853]
                      tunnel: [w846 w853] -> w843
                      tunnel: w841 -> [w845 _]
                      frame "Infected", Default {
                        n758 = case shown="False" w847 {
                          selector: w847 -> [w848 w852]
                          tunnel: [w848 w850] -> w846
                          tunnel: w845 -> [_ w849]
                          frame False {
                            n759 = local write "P9"(w848) -> ()
                          }
                          frame True {
                            n760 = Select(t=w852, s=w849, f=FALSE) -> (s? t:f=w850:bool)
                            n761 = local write "P9"(w850) -> ()
                          }
                        }
                      }
                      frame "Uninfected" {
                        n762 = local write "P9"(w853) -> ()
                      }
                    }
                  }
                  frame "Dead" {
                    w854 = FALSE ("P1")
                    n763 = local write "P9"(w854) -> ()
                  }
                }
                n764 = case shown="\"Alive\", Default" w777 {
                  tunnel: w779 -> [w830 _]
                  tunnel: [w829 w840] -> w775
                  tunnel: w780 -> [w828 _]
                  tunnel: w774 -> [w827 _]
                  frame "Alive", Default {
                    n765 = case shown="\"Uninfected\"" w828 {
                      tunnel: w830 -> [w833 w839]
                      tunnel: [w832 w839] -> w829
                      tunnel: w827 -> [w831 _]
                      frame "Infected", Default {
                        n766 = case shown="False" w833 {
                          selector: w833 -> [w834 w838]
                          tunnel: [w834 w836] -> w832
                          tunnel: w831 -> [_ w835]
                          frame False {
                            n767 = local write "P10"(w834) -> ()
                          }
                          frame True {
                            n768 = Select(t=w838, s=w835, f=FALSE) -> (s? t:f=w836:bool)
                            n769 = local write "P10"(w836) -> ()
                          }
                        }
                      }
                      frame "Uninfected" {
                        n770 = local write "P10"(w839) -> ()
                      }
                    }
                  }
                  frame "Dead" {
                    w840 = FALSE ("P1")
                    n771 = local write "P10"(w840) -> ()
                  }
                }
                n772 = Build Array(w826, w816, w811, w802, w801, w796, w791, w786, w781, w775) -> (w825:bool[])
              }
              frame True {
                n773 = local read "Alive? P10"() -> (w1025:enum16{"Alive", "Dead"})
                n774 = local read "Alive? P7"() -> (w996:enum16{"Alive", "Dead"})
                n775 = local read "Alive? P5"() -> (w990:enum16{"Alive", "Dead"})
                n776 = local read "Alive? P1"() -> (w973:enum16{"Alive", "Dead"})
                n777 = local read "Alive? P2"() -> (w977:enum16{"Alive", "Dead"})
                n778 = local read "Alive? P3"() -> (w981:enum16{"Alive", "Dead"})
                n779 = local read "Alive? P4"() -> (w985:enum16{"Alive", "Dead"})
                n780 = local read "Alive? P9"() -> (w1021:enum16{"Alive", "Dead"})
                n781 = local read "Alive? P8"() -> (w1001:enum16{"Alive", "Dead"})
                n782 = local read "Alive? P6"() -> (w995:enum16{"Alive", "Dead"})
                n783 = Index Array(array=w1004, index=0) -> (element=w968:bool)
                n784 = Index Array(array=w1003, index=0) -> (element=w972:bool)
                n785 = Index Array(array=w1004, index=1) -> (element=w976:bool)
                n786 = Index Array(array=w1003, index=1) -> (element=w975:bool)
                n787 = Index Array(array=w1004, index=2) -> (element=w980:bool)
                n788 = Index Array(array=w1003, index=2) -> (element=w979:bool)
                n789 = Index Array(array=w1004, index=3) -> (element=w984:bool)
                n790 = Index Array(array=w1003, index=3) -> (element=w983:bool)
                n791 = Index Array(array=w1004, index=8) -> (element=w1022:bool)
                n792 = Index Array(array=w1003, index=8) -> (element=w1023:bool)
                n793 = Index Array(array=w1004, index=9) -> (element=w1026:bool)
                n794 = Index Array(array=w1003, index=9) -> (element=w1027:bool)
                n795 = Index Array(array=w1004, index=7) -> (element=w1000:bool)
                n796 = Index Array(array=w1003, index=7) -> (element=w999:bool)
                n797 = Index Array(array=w1004, index=4) -> (element=w992:bool)
                n798 = Index Array(array=w1003, index=4) -> (element=w991:bool)
                n799 = Index Array(array=w1004, index=6) -> (element=w998:bool)
                n800 = Index Array(array=w1003, index=6) -> (element=w997:bool)
                n801 = Index Array(array=w1004, index=5) -> (element=w994:bool)
                n802 = Index Array(array=w1003, index=5) -> (element=w993:bool)
                n803 = case shown="\"Alive\", Default" w977 {
                  tunnel: w975 -> [_ w1074]
                  tunnel: w976 -> [_ w1072]
                  tunnel: [w1065 w1070] -> w974
                  tunnel: w970 -> [_ w1069]
                  tunnel: w969 -> [_ w1068]
                  tunnel: w967 -> [_ w1067]
                  frame "Dead" {
                    w1065 = FALSE ("P10")
                    n804 = local write "Alive? P2"(enum16{"Alive", "Dead"}."Dead") -> ()
                    n805 = local write "P2"(w1065) -> ()
                  }
                  frame "Alive", Default {
                    n806 = And(x=w1072, y=w1074) -> (x .and. y?=w1073:bool)
                    n807 = case shown="True" w1073 {
                      tunnel: w1072 -> [w1076 _]
                      tunnel: [w1076 w1081] -> w1070
                      tunnel: [enum16{"Alive", "Dead"}."Alive" w1080] -> w1071
                      tunnel: w1069 -> [_ w1079]
                      tunnel: w1068 -> [_ w1078]
                      tunnel: w1067 -> [_ w1077]
                      frame False {
                        n808 = local write "P2"(w1076) -> ()
                      }
                      frame True {
                        n809 = Random Number (0-1)() -> (number: 0 to 1=w1083:dbl)
                        n810 = Greater?(x=w1083, y=w1079) -> (0:w1082:bool)
                        n811 = case shown="False" w1082 {
                          tunnel: [w1087 w1090] -> w1081
                          tunnel: [enum16{"Alive", "Dead"}."Alive" w1089] -> w1080
                          tunnel: w1078 -> [_ w1088]
                          tunnel: w1077 -> [w1085 _]
                          frame False {
                            w1087 = FALSE ("P1")
                            # "康復"
                            n812 = local write "P2 Infeted?"(enum16{"Infected", "Uninfected"}."Infected" ("P5 Infeted?")) -> ()
                            n813 = property on="P2" class="Bool (strict)"("Colors [4]"=w1085) -> ()  [unwired: 2 in, 2 out]
                            n814 = local write "P2"(w1087) -> ()
                          }
                          frame True {
                            n815 = Random Number (0-1)() -> (number: 0 to 1=w1092:dbl)
                            n816 = Greater?(x=w1092, y=w1088) -> (0:w1091:bool)
                            n817 = case shown="True" w1091 {
                              tunnel: [w1094 w1096] -> w1090
                              tunnel: [enum16{"Alive", "Dead"}."Dead" enum16{"Alive", "Dead"}."Alive"] -> w1089
                              frame False {
                                w1094 = FALSE ("P1")
                                # "死亡"
                                n818 = property on="P2" class="Bool (strict)"("Value"=w1094, "Visible"=w1094) -> ()  [unwired: 2 in, 2 out]
                              }
                              frame True {
                                w1096 = TRUE ("P1")
                                # "繼續生病"
                                n819 = local write "P2"(w1096) -> ()
                              }
                            }
                          }
                        }
                      }
                    }
                    n820 = local write "Alive? P2"(w1071) -> ()
                  }
                }
                n821 = case shown="\"Alive\", Default" w981 {
                  tunnel: w979 -> [_ w1106]
                  tunnel: w980 -> [_ w1104]
                  tunnel: [w1097 w1102] -> w978
                  tunnel: w970 -> [_ w1101]
                  tunnel: w969 -> [_ w1100]
                  tunnel: w967 -> [_ w1099]
                  frame "Dead" {
                    w1097 = FALSE ("P10")
                    n822 = local write "Alive? P3"(enum16{"Alive", "Dead"}."Dead") -> ()
                    n823 = local write "P3"(w1097) -> ()
                  }
                  frame "Alive", Default {
                    n824 = And(x=w1104, y=w1106) -> (x .and. y?=w1105:bool)
                    n825 = case shown="True" w1105 {
                      tunnel: w1104 -> [w1108 _]
                      tunnel: [w1108 w1113] -> w1102
                      tunnel: [enum16{"Alive", "Dead"}."Alive" w1112] -> w1103
                      tunnel: w1101 -> [_ w1111]
                      tunnel: w1100 -> [_ w1110]
                      tunnel: w1099 -> [_ w1109]
                      frame False {
                        n826 = local write "P3"(w1108) -> ()
                      }
                      frame True {
                        n827 = Random Number (0-1)() -> (number: 0 to 1=w1115:dbl)
                        n828 = Greater?(x=w1115, y=w1111) -> (0:w1114:bool)
                        n829 = case shown="False" w1114 {
                          tunnel: [w1119 w1122] -> w1113
                          tunnel: [enum16{"Alive", "Dead"}."Alive" w1121] -> w1112
                          tunnel: w1110 -> [_ w1120]
                          tunnel: w1109 -> [w1117 _]
                          frame False {
                            w1119 = FALSE ("P1")
                            # "康復"
                            n830 = local write "P3 Infeted?"(enum16{"Infected", "Uninfected"}."Infected" ("P5 Infeted?")) -> ()
                            n831 = property on="P3" class="Bool (strict)"("Colors [4]"=w1117) -> ()  [unwired: 2 in, 2 out]
                            n832 = local write "P3"(w1119) -> ()
                          }
                          frame True {
                            n833 = Random Number (0-1)() -> (number: 0 to 1=w1124:dbl)
                            n834 = Greater?(x=w1124, y=w1120) -> (0:w1123:bool)
                            n835 = case shown="True" w1123 {
                              tunnel: [w1126 w1128] -> w1122
                              tunnel: [enum16{"Alive", "Dead"}."Dead" enum16{"Alive", "Dead"}."Alive"] -> w1121
                              frame False {
                                w1126 = FALSE ("P1")
                                # "死亡"
                                n836 = property on="P3" class="Bool (strict)"("Value"=w1126, "Visible"=w1126) -> ()  [unwired: 2 in, 2 out]
                              }
                              frame True {
                                w1128 = TRUE ("P1")
                                # "繼續生病"
                                n837 = local write "P3"(w1128) -> ()
                              }
                            }
                          }
                        }
                      }
                    }
                    n838 = local write "Alive? P3"(w1103) -> ()
                  }
                }
                n839 = case shown="\"Alive\", Default" w990 {
                  tunnel: w991 -> [_ w1170]
                  tunnel: w992 -> [_ w1168]
                  tunnel: [w1161 w1166] -> w989
                  tunnel: w970 -> [_ w1165]
                  tunnel: w969 -> [_ w1164]
                  tunnel: w967 -> [_ w1163]
                  frame "Dead" {
                    w1161 = FALSE ("P10")
                    n840 = local write "Alive? P5"(enum16{"Alive", "Dead"}."Dead") -> ()
                    n841 = local write "P5"(w1161) -> ()
                  }
                  frame "Alive", Default {
                    n842 = And(x=w1168, y=w1170) -> (x .and. y?=w1169:bool)
                    n843 = case shown="True" w1169 {
                      tunnel: w1168 -> [w1172 _]
                      tunnel: [w1172 w1177] -> w1166
                      tunnel: [enum16{"Alive", "Dead"}."Alive" w1176] -> w1167
                      tunnel: w1165 -> [_ w1175]
                      tunnel: w1164 -> [_ w1174]
                      tunnel: w1163 -> [_ w1173]
                      frame False {
                        n844 = local write "P5"(w1172) -> ()
                      }
                      frame True {
                        n845 = Random Number (0-1)() -> (number: 0 to 1=w1179:dbl)
                        n846 = Greater?(x=w1179, y=w1175) -> (0:w1178:bool)
                        n847 = case shown="False" w1178 {
                          tunnel: [w1183 w1186] -> w1177
                          tunnel: [enum16{"Alive", "Dead"}."Alive" w1185] -> w1176
                          tunnel: w1174 -> [_ w1184]
                          tunnel: w1173 -> [w1181 _]
                          frame False {
                            w1183 = FALSE ("P1")
                            # "康復"
                            n848 = local write "P5 Infeted?"(enum16{"Infected", "Uninfected"}."Infected" ("P5 Infeted?")) -> ()
                            n849 = local write "P5"(w1183) -> ()
                            n850 = property on="P5" class="Bool (strict)"("Colors [4]"=w1181) -> ()  [unwired: 2 in, 2 out]
                          }
                          frame True {
                            n851 = Random Number (0-1)() -> (number: 0 to 1=w1188:dbl)
                            n852 = Greater?(x=w1188, y=w1184) -> (0:w1187:bool)
                            n853 = case shown="True" w1187 {
                              tunnel: [w1190 w1192] -> w1186
                              tunnel: [enum16{"Alive", "Dead"}."Dead" enum16{"Alive", "Dead"}."Alive"] -> w1185
                              frame False {
                                w1190 = FALSE ("P1")
                                # "死亡"
                                n854 = property on="P5" class="Bool (strict)"("Value"=w1190, "Visible"=w1190) -> ()  [unwired: 2 in, 2 out]
                              }
                              frame True {
                                w1192 = TRUE ("P1")
                                # "繼續生病"
                                n855 = local write "P5"(w1192) -> ()
                              }
                            }
                          }
                        }
                      }
                    }
                    n856 = local write "Alive? P5"(w1167) -> ()
                  }
                }
                n857 = case shown="\"Alive\", Default" w1021 {
                  tunnel: w1023 -> [_ w1298]
                  tunnel: w1022 -> [_ w1296]
                  tunnel: [w1289 w1294] -> w1002
                  tunnel: w970 -> [_ w1293]
                  tunnel: w969 -> [_ w1292]
                  tunnel: w967 -> [_ w1291]
                  frame "Dead" {
                    w1289 = FALSE ("P10")
                    n858 = local write "Alive? P9"(enum16{"Alive", "Dead"}."Dead") -> ()
                    n859 = local write "P9"(w1289) -> ()
                  }
                  frame "Alive", Default {
                    n860 = And(x=w1296, y=w1298) -> (x .and. y?=w1297:bool)
                    n861 = case shown="True" w1297 {
                      tunnel: w1296 -> [w1300 _]
                      tunnel: [w1300 w1305] -> w1294
                      tunnel: [enum16{"Alive", "Dead"}."Alive" w1304] -> w1295
                      tunnel: w1293 -> [_ w1303]
                      tunnel: w1292 -> [_ w1302]
                      tunnel: w1291 -> [_ w1301]
                      frame False {
                        n862 = local write "P9"(w1300) -> ()
                      }
                      frame True {
                        n863 = Random Number (0-1)() -> (number: 0 to 1=w1307:dbl)
                        n864 = Greater?(x=w1307, y=w1303) -> (0:w1306:bool)
                        n865 = case shown="False" w1306 {
                          tunnel: [w1311 w1314] -> w1305
                          tunnel: [enum16{"Alive", "Dead"}."Alive" w1313] -> w1304
                          tunnel: w1302 -> [_ w1312]
                          tunnel: w1301 -> [w1309 _]
                          frame False {
                            w1311 = FALSE ("P1")
                            # "康復"
                            n866 = property on="P9" class="Bool (strict)"("Colors [4]"=w1309) -> ()  [unwired: 2 in, 2 out]
                            n867 = local write "P9 Infeted?"(enum16{"Infected", "Uninfected"}."Infected" ("P5 Infeted?")) -> ()
                            n868 = local write "P9"(w1311) -> ()
                          }
                          frame True {
                            n869 = Random Number (0-1)() -> (number: 0 to 1=w1316:dbl)
                            n870 = Greater?(x=w1316, y=w1312) -> (0:w1315:bool)
                            n871 = case shown="True" w1315 {
                              tunnel: [w1318 w1320] -> w1314
                              tunnel: [enum16{"Alive", "Dead"}."Dead" enum16{"Alive", "Dead"}."Alive"] -> w1313
                              frame False {
                                w1318 = FALSE ("P1")
                                # "死亡"
                                n872 = property on="P9" class="Bool (strict)"("Value"=w1318, "Visible"=w1318) -> ()  [unwired: 2 in, 2 out]
                              }
                              frame True {
                                w1320 = TRUE ("P1")
                                # "繼續生病"
                                n873 = local write "P9"(w1320) -> ()
                              }
                            }
                          }
                        }
                      }
                    }
                    n874 = local write "Alive? P9"(w1295) -> ()
                  }
                }
                n875 = case shown="\"Alive\", Default" w1025 {
                  tunnel: w1027 -> [_ w1330]
                  tunnel: w1026 -> [_ w1328]
                  tunnel: [w1321 w1326] -> w1024
                  tunnel: w970 -> [_ w1325]
                  tunnel: w969 -> [_ w1324]
                  tunnel: w967 -> [_ w1323]
                  frame "Dead" {
                    w1321 = FALSE ("P1")
                    n876 = local write "Alive? P10"(enum16{"Alive", "Dead"}."Dead") -> ()
                    n877 = local write "P10"(w1321) -> ()
                  }
                  frame "Alive", Default {
                    n878 = And(x=w1328, y=w1330) -> (x .and. y?=w1329:bool)
                    n879 = case shown="True" w1329 {
                      tunnel: w1328 -> [w1332 _]
                      tunnel: [w1332 w1337] -> w1326
                      tunnel: [enum16{"Alive", "Dead"}."Alive" w1336] -> w1327
                      tunnel: w1325 -> [_ w1335]
                      tunnel: w1324 -> [_ w1334]
                      tunnel: w1323 -> [_ w1333]
                      frame False {
                        n880 = local write "P10"(w1332) -> ()
                      }
                      frame True {
                        n881 = Random Number (0-1)() -> (number: 0 to 1=w1339:dbl)
                        n882 = Greater?(x=w1339, y=w1335) -> (0:w1338:bool)
                        n883 = case shown="False" w1338 {
                          tunnel: [w1343 w1346] -> w1337
                          tunnel: [enum16{"Alive", "Dead"}."Alive" w1345] -> w1336
                          tunnel: w1334 -> [_ w1344]
                          tunnel: w1333 -> [w1341 _]
                          frame False {
                            w1343 = FALSE ("P1")
                            # "康復"
                            n884 = property on="P10" class="Bool (strict)"("Colors [4]"=w1341) -> ()  [unwired: 2 in, 2 out]
                            n885 = local write "P10 Infeted"(enum16{"Infected", "Uninfected"}."Infected" ("P5 Infeted?")) -> ()
                            n886 = local write "P10"(w1343) -> ()
                          }
                          frame True {
                            n887 = Random Number (0-1)() -> (number: 0 to 1=w1348:dbl)
                            n888 = Greater?(x=w1348, y=w1344) -> (0:w1347:bool)
                            n889 = case shown="True" w1347 {
                              tunnel: [w1350 w1352] -> w1346
                              tunnel: [enum16{"Alive", "Dead"}."Dead" enum16{"Alive", "Dead"}."Alive"] -> w1345
                              frame False {
                                w1350 = FALSE ("P1")
                                # "死亡"
                                n890 = property on="P10" class="Bool (strict)"("Value"=w1350, "Visible"=w1350) -> ()  [unwired: 2 in, 2 out]
                              }
                              frame True {
                                w1352 = TRUE ("P1")
                                # "繼續生病"
                                n891 = local write "P10"(w1352) -> ()
                              }
                            }
                          }
                        }
                      }
                    }
                    n892 = local write "Alive? P10"(w1327) -> ()
                  }
                }
                n893 = case shown="\"Alive\", Default" w973 {
                  tunnel: w972 -> [_ w1042]
                  tunnel: w968 -> [_ w1040]
                  tunnel: [w1033 w1038] -> w971
                  tunnel: w970 -> [_ w1037]
                  tunnel: w969 -> [_ w1036]
                  tunnel: w967 -> [_ w1035]
                  frame "Dead" {
                    w1033 = FALSE ("P10")
                    # "已死亡"
                    n894 = local write "Alive? P1"(enum16{"Alive", "Dead"}."Dead") -> ()
                    n895 = local write "P1"(w1033) -> ()
                  }
                  frame "Alive", Default {
                    n896 = And(x=w1040, y=w1042) -> (x .and. y?=w1041:bool)
                    n897 = case shown="False" w1041 {
                      tunnel: w1040 -> [w1044 _]
                      tunnel: [w1044 w1049] -> w1038
                      tunnel: [enum16{"Alive", "Dead"}."Alive" w1048] -> w1039
                      tunnel: w1037 -> [_ w1047]
                      tunnel: w1036 -> [_ w1046]
                      tunnel: w1035 -> [_ w1045]
                      frame False {
                        # "維持原狀態"
                        n898 = local write "P1"(w1044) -> ()
                      }
                      frame True {
                        n899 = Random Number (0-1)() -> (number: 0 to 1=w1051:dbl)
                        n900 = Greater?(x=w1051, y=w1047) -> (0:w1050:bool)
                        n901 = case shown="False" w1050 {
                          tunnel: [w1055 w1058] -> w1049
                          tunnel: [enum16{"Alive", "Dead"}."Alive" w1057] -> w1048
                          tunnel: w1046 -> [_ w1056]
                          tunnel: w1045 -> [w1053 _]
                          frame False {
                            w1055 = FALSE ("P1")
                            # "康復"
                            n902 = local write "P1 Infeted?"(enum16{"Infected", "Uninfected"}."Infected" ("P5 Infeted?")) -> ()
                            n903 = property on="P1" class="Bool (strict)"("Colors [4]"=w1053) -> ()  [unwired: 2 in, 2 out]
                            n904 = local write "P1"(w1055) -> ()
                          }
                          frame True {
                            n905 = Random Number (0-1)() -> (number: 0 to 1=w1060:dbl)
                            n906 = Greater?(x=w1060, y=w1056) -> (0:w1059:bool)
                            n907 = case shown="True" w1059 {
                              tunnel: [w1062 w1064] -> w1058
                              tunnel: [enum16{"Alive", "Dead"}."Dead" enum16{"Alive", "Dead"}."Alive"] -> w1057
                              frame False {
                                w1062 = FALSE ("P1")
                                # "死亡"
                                n908 = property on="P1" class="Bool (strict)"("Value"=w1062, "Visible"=w1062) -> ()  [unwired: 2 in, 2 out]
                              }
                              frame True {
                                w1064 = TRUE ("P1")
                                # "繼續生病"
                                n909 = local write "P1"(w1064) -> ()
                              }
                            }
                          }
                        }
                      }
                    }
                    n910 = local write "Alive? P1"(w1039) -> ()
                  }
                }
                n911 = case shown="\"Alive\", Default" w985 {
                  tunnel: w983 -> [_ w1138]
                  tunnel: w984 -> [_ w1136]
                  tunnel: [w1129 w1134] -> w982
                  tunnel: w970 -> [_ w1133]
                  tunnel: w969 -> [_ w1132]
                  tunnel: w967 -> [_ w1131]
                  frame "Dead" {
                    w1129 = FALSE ("P10")
                    n912 = local write "Alive? P4"(enum16{"Alive", "Dead"}."Dead") -> ()
                    n913 = local write "P4"(w1129) -> ()
                  }
                  frame "Alive", Default {
                    n914 = And(x=w1136, y=w1138) -> (x .and. y?=w1137:bool)
                    n915 = case shown="True" w1137 {
                      tunnel: w1136 -> [w1140 _]
                      tunnel: [w1140 w1145] -> w1134
                      tunnel: [enum16{"Alive", "Dead"}."Alive" w1144] -> w1135
                      tunnel: w1133 -> [_ w1143]
                      tunnel: w1132 -> [_ w1142]
                      tunnel: w1131 -> [_ w1141]
                      frame False {
                        n916 = local write "P4"(w1140) -> ()
                      }
                      frame True {
                        n917 = Random Number (0-1)() -> (number: 0 to 1=w1147:dbl)
                        n918 = Greater?(x=w1147, y=w1143) -> (0:w1146:bool)
                        n919 = case shown="False" w1146 {
                          tunnel: [w1151 w1154] -> w1145
                          tunnel: [enum16{"Alive", "Dead"}."Alive" w1153] -> w1144
                          tunnel: w1142 -> [_ w1152]
                          tunnel: w1141 -> [w1149 _]
                          frame False {
                            w1151 = FALSE ("P1")
                            # "康復"
                            n920 = local write "P4 Infeted?"(enum16{"Infected", "Uninfected"}."Infected" ("P5 Infeted?")) -> ()
                            n921 = property on="P4" class="Bool (strict)"("Colors [4]"=w1149) -> ()  [unwired: 2 in, 2 out]
                            n922 = local write "P4"(w1151) -> ()
                          }
                          frame True {
                            n923 = Random Number (0-1)() -> (number: 0 to 1=w1156:dbl)
                            n924 = Greater?(x=w1156, y=w1152) -> (0:w1155:bool)
                            n925 = case shown="True" w1155 {
                              tunnel: [w1158 w1160] -> w1154
                              tunnel: [enum16{"Alive", "Dead"}."Dead" enum16{"Alive", "Dead"}."Alive"] -> w1153
                              frame False {
                                w1158 = FALSE ("P1")
                                # "死亡"
                                n926 = property on="P4" class="Bool (strict)"("Value"=w1158, "Visible"=w1158) -> ()  [unwired: 2 in, 2 out]
                              }
                              frame True {
                                w1160 = TRUE ("P1")
                                # "繼續生病"
                                n927 = local write "P4"(w1160) -> ()
                              }
                            }
                          }
                        }
                      }
                    }
                    n928 = local write "Alive? P4"(w1135) -> ()
                  }
                }
                n929 = case shown="\"Alive\", Default" w1001 {
                  tunnel: w999 -> [_ w1266]
                  tunnel: w1000 -> [_ w1264]
                  tunnel: [w1257 w1262] -> w988
                  tunnel: w970 -> [_ w1261]
                  tunnel: w969 -> [_ w1260]
                  tunnel: w967 -> [_ w1259]
                  frame "Dead" {
                    w1257 = FALSE ("P10")
                    n930 = local write "Alive? P8"(enum16{"Alive", "Dead"}."Dead") -> ()
                    n931 = property on="P8" class="Bool (strict)"("Value"=w1257) -> ()  [unwired: 2 in, 2 out]
                  }
                  frame "Alive", Default {
                    n932 = And(x=w1264, y=w1266) -> (x .and. y?=w1265:bool)
                    n933 = case shown="True" w1265 {
                      tunnel: w1264 -> [w1268 _]
                      tunnel: [w1268 w1273] -> w1262
                      tunnel: [enum16{"Alive", "Dead"}."Alive" w1272] -> w1263
                      tunnel: w1261 -> [_ w1271]
                      tunnel: w1260 -> [_ w1270]
                      tunnel: w1259 -> [_ w1269]
                      frame False {
                        n934 = local write "P8"(w1268) -> ()
                      }
                      frame True {
                        n935 = Random Number (0-1)() -> (number: 0 to 1=w1275:dbl)
                        n936 = Greater?(x=w1275, y=w1271) -> (0:w1274:bool)
                        n937 = case shown="False" w1274 {
                          tunnel: [w1279 w1282] -> w1273
                          tunnel: [enum16{"Alive", "Dead"}."Alive" w1281] -> w1272
                          tunnel: w1270 -> [_ w1280]
                          tunnel: w1269 -> [w1277 _]
                          frame False {
                            w1279 = FALSE ("P1")
                            # "康復"
                            n938 = local write "P8 Infeted?"(enum16{"Infected", "Uninfected"}."Infected" ("P5 Infeted?")) -> ()
                            n939 = property on="P8" class="Bool (strict)"("Colors [4]"=w1277) -> ()  [unwired: 2 in, 2 out]
                            n940 = local write "P8"(w1279) -> ()
                          }
                          frame True {
                            n941 = Random Number (0-1)() -> (number: 0 to 1=w1284:dbl)
                            n942 = Greater?(x=w1284, y=w1280) -> (0:w1283:bool)
                            n943 = case shown="True" w1283 {
                              tunnel: [w1286 w1288] -> w1282
                              tunnel: [enum16{"Alive", "Dead"}."Dead" enum16{"Alive", "Dead"}."Alive"] -> w1281
                              frame False {
                                w1286 = FALSE ("P1")
                                # "死亡"
                                n944 = property on="P8" class="Bool (strict)"("Value"=w1286, "Visible"=w1286) -> ()  [unwired: 2 in, 2 out]
                              }
                              frame True {
                                w1288 = TRUE ("P1")
                                # "繼續生病"
                                n945 = local write "P8"(w1288) -> ()
                              }
                            }
                          }
                        }
                      }
                    }
                    n946 = local write "Alive? P8"(w1263) -> ()
                  }
                }
                n947 = case shown="\"Alive\", Default" w995 {
                  tunnel: w993 -> [_ w1202]
                  tunnel: w994 -> [_ w1200]
                  tunnel: [w1193 w1198] -> w986
                  tunnel: w970 -> [_ w1197]
                  tunnel: w969 -> [_ w1196]
                  tunnel: w967 -> [_ w1195]
                  frame "Dead" {
                    w1193 = FALSE ("P10")
                    n948 = local write "Alive? P6"(enum16{"Alive", "Dead"}."Dead") -> ()
                    n949 = local write "P6"(w1193) -> ()
                  }
                  frame "Alive", Default {
                    n950 = And(x=w1200, y=w1202) -> (x .and. y?=w1201:bool)
                    n951 = case shown="True" w1201 {
                      tunnel: w1200 -> [w1204 _]
                      tunnel: [w1204 w1209] -> w1198
                      tunnel: [enum16{"Alive", "Dead"}."Alive" w1208] -> w1199
                      tunnel: w1197 -> [_ w1207]
                      tunnel: w1196 -> [_ w1206]
                      tunnel: w1195 -> [_ w1205]
                      frame False {
                        n952 = local write "P6"(w1204) -> ()
                      }
                      frame True {
                        n953 = Random Number (0-1)() -> (number: 0 to 1=w1211:dbl)
                        n954 = Greater?(x=w1211, y=w1207) -> (0:w1210:bool)
                        n955 = case shown="False" w1210 {
                          tunnel: [w1215 w1218] -> w1209
                          tunnel: [enum16{"Alive", "Dead"}."Alive" w1217] -> w1208
                          tunnel: w1206 -> [_ w1216]
                          tunnel: w1205 -> [w1213 _]
                          frame False {
                            w1215 = FALSE ("P1")
                            # "康復"
                            n956 = property on="P6" class="Bool (strict)"("Colors [4]"=w1213) -> ()  [unwired: 2 in, 2 out]
                            n957 = local write "P6 Infeted?"(enum16{"Infected", "Uninfected"}."Infected" ("P5 Infeted?")) -> ()
                            n958 = local write "P6"(w1215) -> ()
                          }
                          frame True {
                            n959 = Random Number (0-1)() -> (number: 0 to 1=w1220:dbl)
                            n960 = Greater?(x=w1220, y=w1216) -> (0:w1219:bool)
                            n961 = case shown="True" w1219 {
                              tunnel: [w1222 w1224] -> w1218
                              tunnel: [enum16{"Alive", "Dead"}."Dead" enum16{"Alive", "Dead"}."Alive"] -> w1217
                              frame False {
                                w1222 = FALSE ("P1")
                                # "死亡"
                                n962 = property on="P6" class="Bool (strict)"("Value"=w1222, "Visible"=w1222) -> ()  [unwired: 2 in, 2 out]
                              }
                              frame True {
                                w1224 = TRUE ("P1")
                                # "繼續生病"
                                n963 = local write "P6"(w1224) -> ()
                              }
                            }
                          }
                        }
                      }
                    }
                    n964 = local write "Alive? P6"(w1199) -> ()
                  }
                }
                n965 = case shown="\"Alive\", Default" w996 {
                  tunnel: w997 -> [_ w1234]
                  tunnel: w998 -> [_ w1232]
                  tunnel: [w1225 w1230] -> w987
                  tunnel: w970 -> [_ w1229]
                  tunnel: w969 -> [_ w1228]
                  tunnel: w967 -> [_ w1227]
                  frame "Dead" {
                    w1225 = FALSE ("P10")
                    n966 = local write "Alive? P7"(enum16{"Alive", "Dead"}."Dead") -> ()
                    n967 = local write "P7"(w1225) -> ()
                  }
                  frame "Alive", Default {
                    n968 = And(x=w1232, y=w1234) -> (x .and. y?=w1233:bool)
                    n969 = case shown="True" w1233 {
                      tunnel: w1232 -> [w1236 _]
                      tunnel: [w1236 w1241] -> w1230
                      tunnel: [enum16{"Alive", "Dead"}."Alive" w1240] -> w1231
                      tunnel: w1229 -> [_ w1239]
                      tunnel: w1228 -> [_ w1238]
                      tunnel: w1227 -> [_ w1237]
                      frame False {
                        n970 = local write "P7"(w1236) -> ()
                      }
                      frame True {
                        n971 = Random Number (0-1)() -> (number: 0 to 1=w1243:dbl)
                        n972 = Greater?(x=w1243, y=w1239) -> (0:w1242:bool)
                        n973 = case shown="False" w1242 {
                          tunnel: [w1247 w1250] -> w1241
                          tunnel: [enum16{"Alive", "Dead"}."Alive" w1249] -> w1240
                          tunnel: w1238 -> [_ w1248]
                          tunnel: w1237 -> [w1245 _]
                          frame False {
                            w1247 = FALSE ("P1")
                            # "康復"
                            n974 = local write "P7 Infeted?"(enum16{"Infected", "Uninfected"}."Infected" ("P5 Infeted?")) -> ()
                            n975 = property on="P7" class="Bool (strict)"("Colors [4]"=w1245) -> ()  [unwired: 2 in, 2 out]
                            n976 = local write "P7"(w1247) -> ()
                          }
                          frame True {
                            n977 = Random Number (0-1)() -> (number: 0 to 1=w1252:dbl)
                            n978 = Greater?(x=w1252, y=w1248) -> (0:w1251:bool)
                            n979 = case shown="True" w1251 {
                              tunnel: [w1254 w1256] -> w1250
                              tunnel: [enum16{"Alive", "Dead"}."Dead" enum16{"Alive", "Dead"}."Alive"] -> w1249
                              frame False {
                                w1254 = FALSE ("P1")
                                # "死亡"
                                n980 = property on="P7" class="Bool (strict)"("Value"=w1254, "Visible"=w1254) -> ()  [unwired: 2 in, 2 out]
                              }
                              frame True {
                                w1256 = TRUE ("P1")
                                # "繼續生病"
                                n981 = local write "P7"(w1256) -> ()
                              }
                            }
                          }
                        }
                      }
                    }
                    n982 = local write "Alive? P7"(w1231) -> ()
                  }
                }
                n983 = Build Array(w971, w974, w978, w982, w989, w986, w987, w988, w1002, w1024) -> (w1030:bool[])
              }
            }
            n984 = case shown="True" w766 {
              tunnel: [w772 w773] -> w765
              tunnel: w761 -> [w772 _]
              tunnel: w760 -> [_ w773]
              frame False {
              }
              frame True {
              }
            }
          }
          frame #2 {
            n985 = local read "Alive? P1"() -> (w1379:enum16{"Alive", "Dead"})
            n986 = local read "Alive? P2"() -> (w1378:enum16{"Alive", "Dead"})
            n987 = local read "Alive? P3"() -> (w1377:enum16{"Alive", "Dead"})
            n988 = local read "Alive? P4"() -> (w1374:enum16{"Alive", "Dead"})
            n989 = local read "Alive? P5"() -> (w1375:enum16{"Alive", "Dead"})
            n990 = local read "Alive? P8"() -> (w1373:enum16{"Alive", "Dead"})
            n991 = local read "Alive? P10"() -> (w1371:enum16{"Alive", "Dead"})
            n992 = local read "Alive? P6"() -> (w1376:enum16{"Alive", "Dead"})
            n993 = local read "Alive? P7"() -> (w1360:enum16{"Alive", "Dead"})
            n994 = local read "Alive? P9"() -> (w1372:enum16{"Alive", "Dead"})
            n995 = case shown="\"Alive\", Default" w1379 {
              tunnel: [w1428 3.0 ("f")] -> w1370
              frame "Alive", Default {
                n996 = local read "P1"() -> (w1430:bool)
                n997 = Select(t=1.0, s=w1430, f=2.0) -> (s? t:f=w1428:dbl)
              }
              frame "Dead" {
              }
            }
            n998 = case shown="\"Alive\", Default" w1378 {
              tunnel: [w1423 3.0 ("f")] -> w1369
              frame "Alive", Default {
                n999 = local read "P2"() -> (w1425:bool)
                n1000 = Select(t=1.0, s=w1425, f=2.0) -> (s? t:f=w1423:dbl)
              }
              frame "Dead" {
              }
            }
            n1001 = case shown="\"Alive\", Default" w1377 {
              tunnel: [w1418 3.0 ("f")] -> w1368
              frame "Alive", Default {
                n1002 = local read "P3"() -> (w1420:bool)
                n1003 = Select(t=1.0, s=w1420, f=2.0) -> (s? t:f=w1418:dbl)
              }
              frame "Dead" {
              }
            }
            n1004 = case shown="\"Alive\", Default" w1374 {
              tunnel: [w1413 3.0 ("f")] -> w1367
              frame "Alive", Default {
                n1005 = local read "P4"() -> (w1415:bool)
                n1006 = Select(t=1.0, s=w1415, f=2.0) -> (s? t:f=w1413:dbl)
              }
              frame "Dead" {
              }
            }
            n1007 = case shown="\"Alive\", Default" w1375 {
              tunnel: [w1408 3.0 ("f")] -> w1366
              frame "Alive", Default {
                n1008 = local read "P5"() -> (w1410:bool)
                n1009 = Select(t=1.0, s=w1410, f=2.0) -> (s? t:f=w1408:dbl)
              }
              frame "Dead" {
              }
            }
            n1010 = case shown="\"Alive\", Default" w1360 {
              tunnel: [w1383 3.0 ("f")] -> w1356
              frame "Alive", Default {
                n1011 = local read "P7"() -> (w1385:bool)
                n1012 = Select(t=1.0, s=w1385, f=2.0) -> (s? t:f=w1383:dbl)
              }
              frame "Dead" {
              }
            }
            n1013 = case shown="\"Alive\", Default" w1373 {
              tunnel: [w1398 3.0 ("f")] -> w1357
              frame "Alive", Default {
                n1014 = local read "P8"() -> (w1400:bool)
                n1015 = Select(t=1.0, s=w1400, f=2.0) -> (s? t:f=w1398:dbl)
              }
              frame "Dead" {
              }
            }
            n1016 = case shown="\"Alive\", Default" w1376 {
              tunnel: [w1403 3.0 ("f")] -> w1365
              frame "Alive", Default {
                n1017 = local read "P6"() -> (w1405:bool)
                n1018 = Select(t=1.0, s=w1405, f=2.0) -> (s? t:f=w1403:dbl)
              }
              frame "Dead" {
              }
            }
            n1019 = case shown="\"Alive\", Default" w1372 {
              tunnel: [w1393 3.0 ("f")] -> w1358
              frame "Alive", Default {
                n1020 = local read "P9"() -> (w1395:bool)
                n1021 = Select(t=1.0, s=w1395, f=2.0) -> (s? t:f=w1393:dbl)
              }
              frame "Dead" {
              }
            }
            n1022 = case shown="\"Alive\", Default" w1371 {
              tunnel: [w1388 3.0 ("f")] -> w1359
              frame "Alive", Default {
                n1023 = local read "P10"() -> (w1390:bool)
                n1024 = Select(t=1.0, s=w1390, f=2.0) -> (s? t:f=w1388:dbl)
              }
              frame "Dead" {
              }
            }
            n1025 = Build Array(w1370, w1369, w1368, w1367, w1366, w1365, w1356, w1357, w1358, w1359) -> (w1364:dbl[])
            n1026 = call "Status Count.vi"("Status"=w1364) -> ("Dead"=w1363:i32, "Helathy"=w1362:i32, "Infected"=w1361:i32)
            n1027 = Build Array(w1363, w1362, w1361) -> (w1354:i32[])
            n1028 = call-poly <vilib>:"Plot Helper.vi"("offset vector"=sgl[] [0.0, 0.0, 0.0], "x vector"=w1354) -> ("3D Plot lvclass Array out"=→"3D Pie":refnum<class "3D Plot Datatype.lvclass">[])  [unwired: 1 in, 8 out]
          }
        }
        "Numeric" <- w89
      }
    }
  }
